vi "Turbulence_3.0_LevelResistors.vi"() -> ()   [LabVIEW 2018]
uses:
  Quantum Composers 9000 Series.lvlib
  LightField Automation.lvclass
  Mercury iXX.lvlib
  Temperature (Read).vi
  Temperature.lvlib
  Open Temperature Device.vi
  Comms Transport Layer.ctl
  Keithley 2600 Series.lvlib
  Channel.ctl
  DAQmx Read (Counter DBL 1Chan 1Samp).vi
  Catalogue (Read).vi
  System.lvlib
  Open System.vi
panel:
  in  "3He Check":bool
  out "MFC Error Out":errorcluster
  out "Lakeshore218 Error":errorcluster
  in  "File Exists":bool
  out "Log":refnum<file>
  in  "Motor free":bool
  in  "RESTART":bool
  out "time string":string
  out "Timestamp":string
  out "Log Error":errorcluster
  in  "CLOSE":bool
  in  "RECORD":bool
  in  "Turbulence":T1(tab)
  in  "# Frames":i32=1000 min=0 step=1
  in  "New Background Movie":bool
  in  "On CCD Acc.":i32=3 min=0 step=1
  in  "Cycle time\n(ms)":i32=3 min=0 step=1
  out "High Level\n(Ohms)":dbl format="%.1f"
  out "Low Level\n(Ohms)":dbl format="%.1f"
  in  "New Background Frame":bool
  out "Rate (Hz)":dbl
  out "Incident":dbl
  in  "BIN":u16(ring)=2 items=["1x1", "2x2", "4x4"]
  in  "MODE":u16(ring) items=["Normal", "DIF"]
  in  "Enable":bool
  out "Rate (Hz)":dbl
  out "Detected":dbl
  in  "Script\nEnd":u32=1 step=1
  in  "Sample Space Pump":bool
  in  "Siphon Pump":bool
  in  "Neutron Shutter":bool
  in  "Manual Script Entry (0)":string
  in  "READY":bool
  out "Power (mW)":dbl format="%_3f"
  out "Tank Pressure 2 (Torr)":string="0.0"
  in  "LIGHTFIELD":bool
  in  "SCRIPTING":bool
  in  "Top Coil":bool
  out "Tank Pressure 1 (Torr)":string="0.0"
  out "Cell (K)":dbl format="%.3f"
  out "Cryostat (K)":dbl format="%.3f"
  in  "Data Interval (s)":dbl=0.5 min=0.4 max=10.0 step=0.05
  in  "RUN/STOP":bool
  in  "Bottom Coil":bool
  in  "Bottom Coil (mA)":dbl min=-1000.0 max=1000.0 step=1e-05
  in  "Top Coil (mA)":dbl min=-1000.0 max=1000.0 step=1e-05
  in  "Percent Open":i32 min=0 max=100 step=5
  in  "COOLDOWN":bool
  in  "Script\n#":i32 step=1
  in  "Kill Switch":bool
  in  "DATA":bool
  out "Scripting \nError":T2
  in  "Shutter Mode":u16(ring)=1 items=["Manual"=1, "XGate"=5]
  in  "Time (s)":i32=120 min=1 max=300 step=1
  in  "REFILL":bool
  in  "AUTOFILL":bool
  in  "LL (Ohms)":dbl=900.0 min=750.0 max=15000.0 step=1.0
  in  "HL (Ohms)":dbl=900.0 min=750.0 max=15000.0 step=1.0
  in  "Fill":bool
  in  "Tare":bool
  out "Actual 3He\nTank Pressure":dbl min=0.0 max=100.0 step=5.0 format="%#.1g"
  out "Desired V2\nPressure (3He)":dbl min=0.0 max=100.0 step=5.0 format="%#.1f"
  in  "Desired Tank\nPressure (3He)":dbl min=0.0 max=100.0 step=0.01 format="%#.2f"
  in  "Log Pressure":bool
  out "4He Pressure (Torr)":string="-0.1"
  out "3He Pressure (Torr)":string="1"
  in  "Fill Time (s)":u32=10
  out "Temperature Error":errorcluster={"status"=TRUE, "code"=-1073807339, "source"="VISA Read in Mercury iXX.lvlib:Query (Dynamic).vit->Mercury iXX.lvlib:Query (Low Level).vi:10049->Mercury iXX.lvlib:Query.vi:3960048->Mercury iXX.lvlib:Read (Str).vi:5300004->Mercury iXX.lvlib:System.lvlib:Catalogue (Read).vi->Turbulence.vi"}
  out "File I/O Error":errorcluster
  out "4He Gauge Error":errorcluster={"status"=TRUE, "code"=-1073807343, "source"="VISA Open in Turbulence.vi"}
  out "Heater Error":errorcluster={"status"=FALSE, "code"=1073676293, "source"="VISA Read in Keithley 2600 Series.lvlib:Print Number.vi->Keithley 2600 Series.lvlib:Measure.vi->Turbulence.vi"}
  out "Pulse Generator Error":errorcluster
  out "3He Gauge Error":errorcluster={"status"=FALSE, "code"=1073676293, "source"="VISA Read in 3HeClose.vi->Turbulence.vi"}
  out "Relay Errror":errorcluster
  out "Zaber Motor Error":errorcluster
  out "LightField Error":errorcluster
  out "Shutter Error":errorcluster
  # "Camera Controls"
  # "Temperature Readout"
  # "Pressure Readout"
  # "Neutron Counts"
  # "Automation"
  # "Heater Controls"
  # "Relay Controls"
  # "Needle Valve Control"
  # "Neutron Shutter"
  # "Optical Shutter"
  # "Siphon Pump"
  # "Laser Power Meter"
  # "Sample Space\nPump"
  # "V1 = 4075 mL"
  # "V2 = 15.5 mL"
  # "V3 = 78.8 mL"
  # "Quartz\nCell"
  # "4"
  # "3psi relief"
  # "MFC"
  # "V1"
  # "4L Tank"
  # "Turbo Pump"
  # "V2"
  # "V3"
  # "3"
  # "10psi relief"
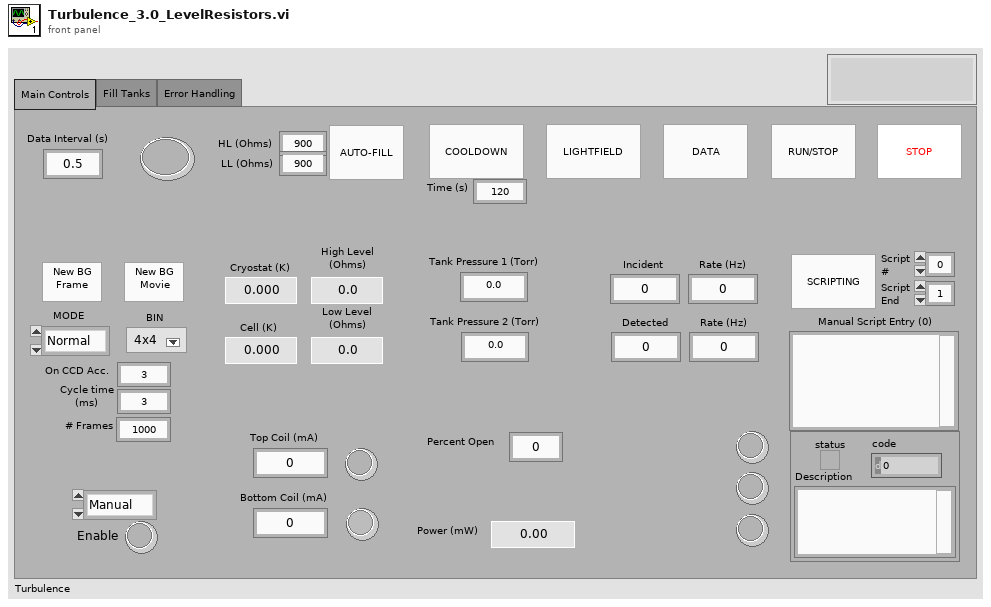
[diagram p1: front panel]
types:
  T1 = enum32{"Main Controls", "Fill Tanks", "Error Handling"}
  T2 = cluster{"status":bool, "code":i32, "Description":string}
  T3 = typedef "Mercury iXX.lvlib/Comms Transport Layer.ctl" = enum16{"Ethernet TCP/IP", "USB", "ISOBus - RS-232", "GPIB"}
  T4 = typedef "Mercury iXX.lvlib/Mercury Reference.ctl" = cluster{"Comms":refnum<visa-resource-name>, "Device ID":string[], "Comms Layer":T3, "Command":string, "Query reference":T5}
  T5 = typedef "Mercury iXX.lvlib/Query Dynamic Reference.ctl" = refnum<vi>
  T6 = enum32{"Current", "Voltage", "IV", "Resistance", "Power"}
  T7 = typedef "Keithley 2600 Series.lvlib/Channel.ctl" = enum32{"Channel A", "Channel B"}
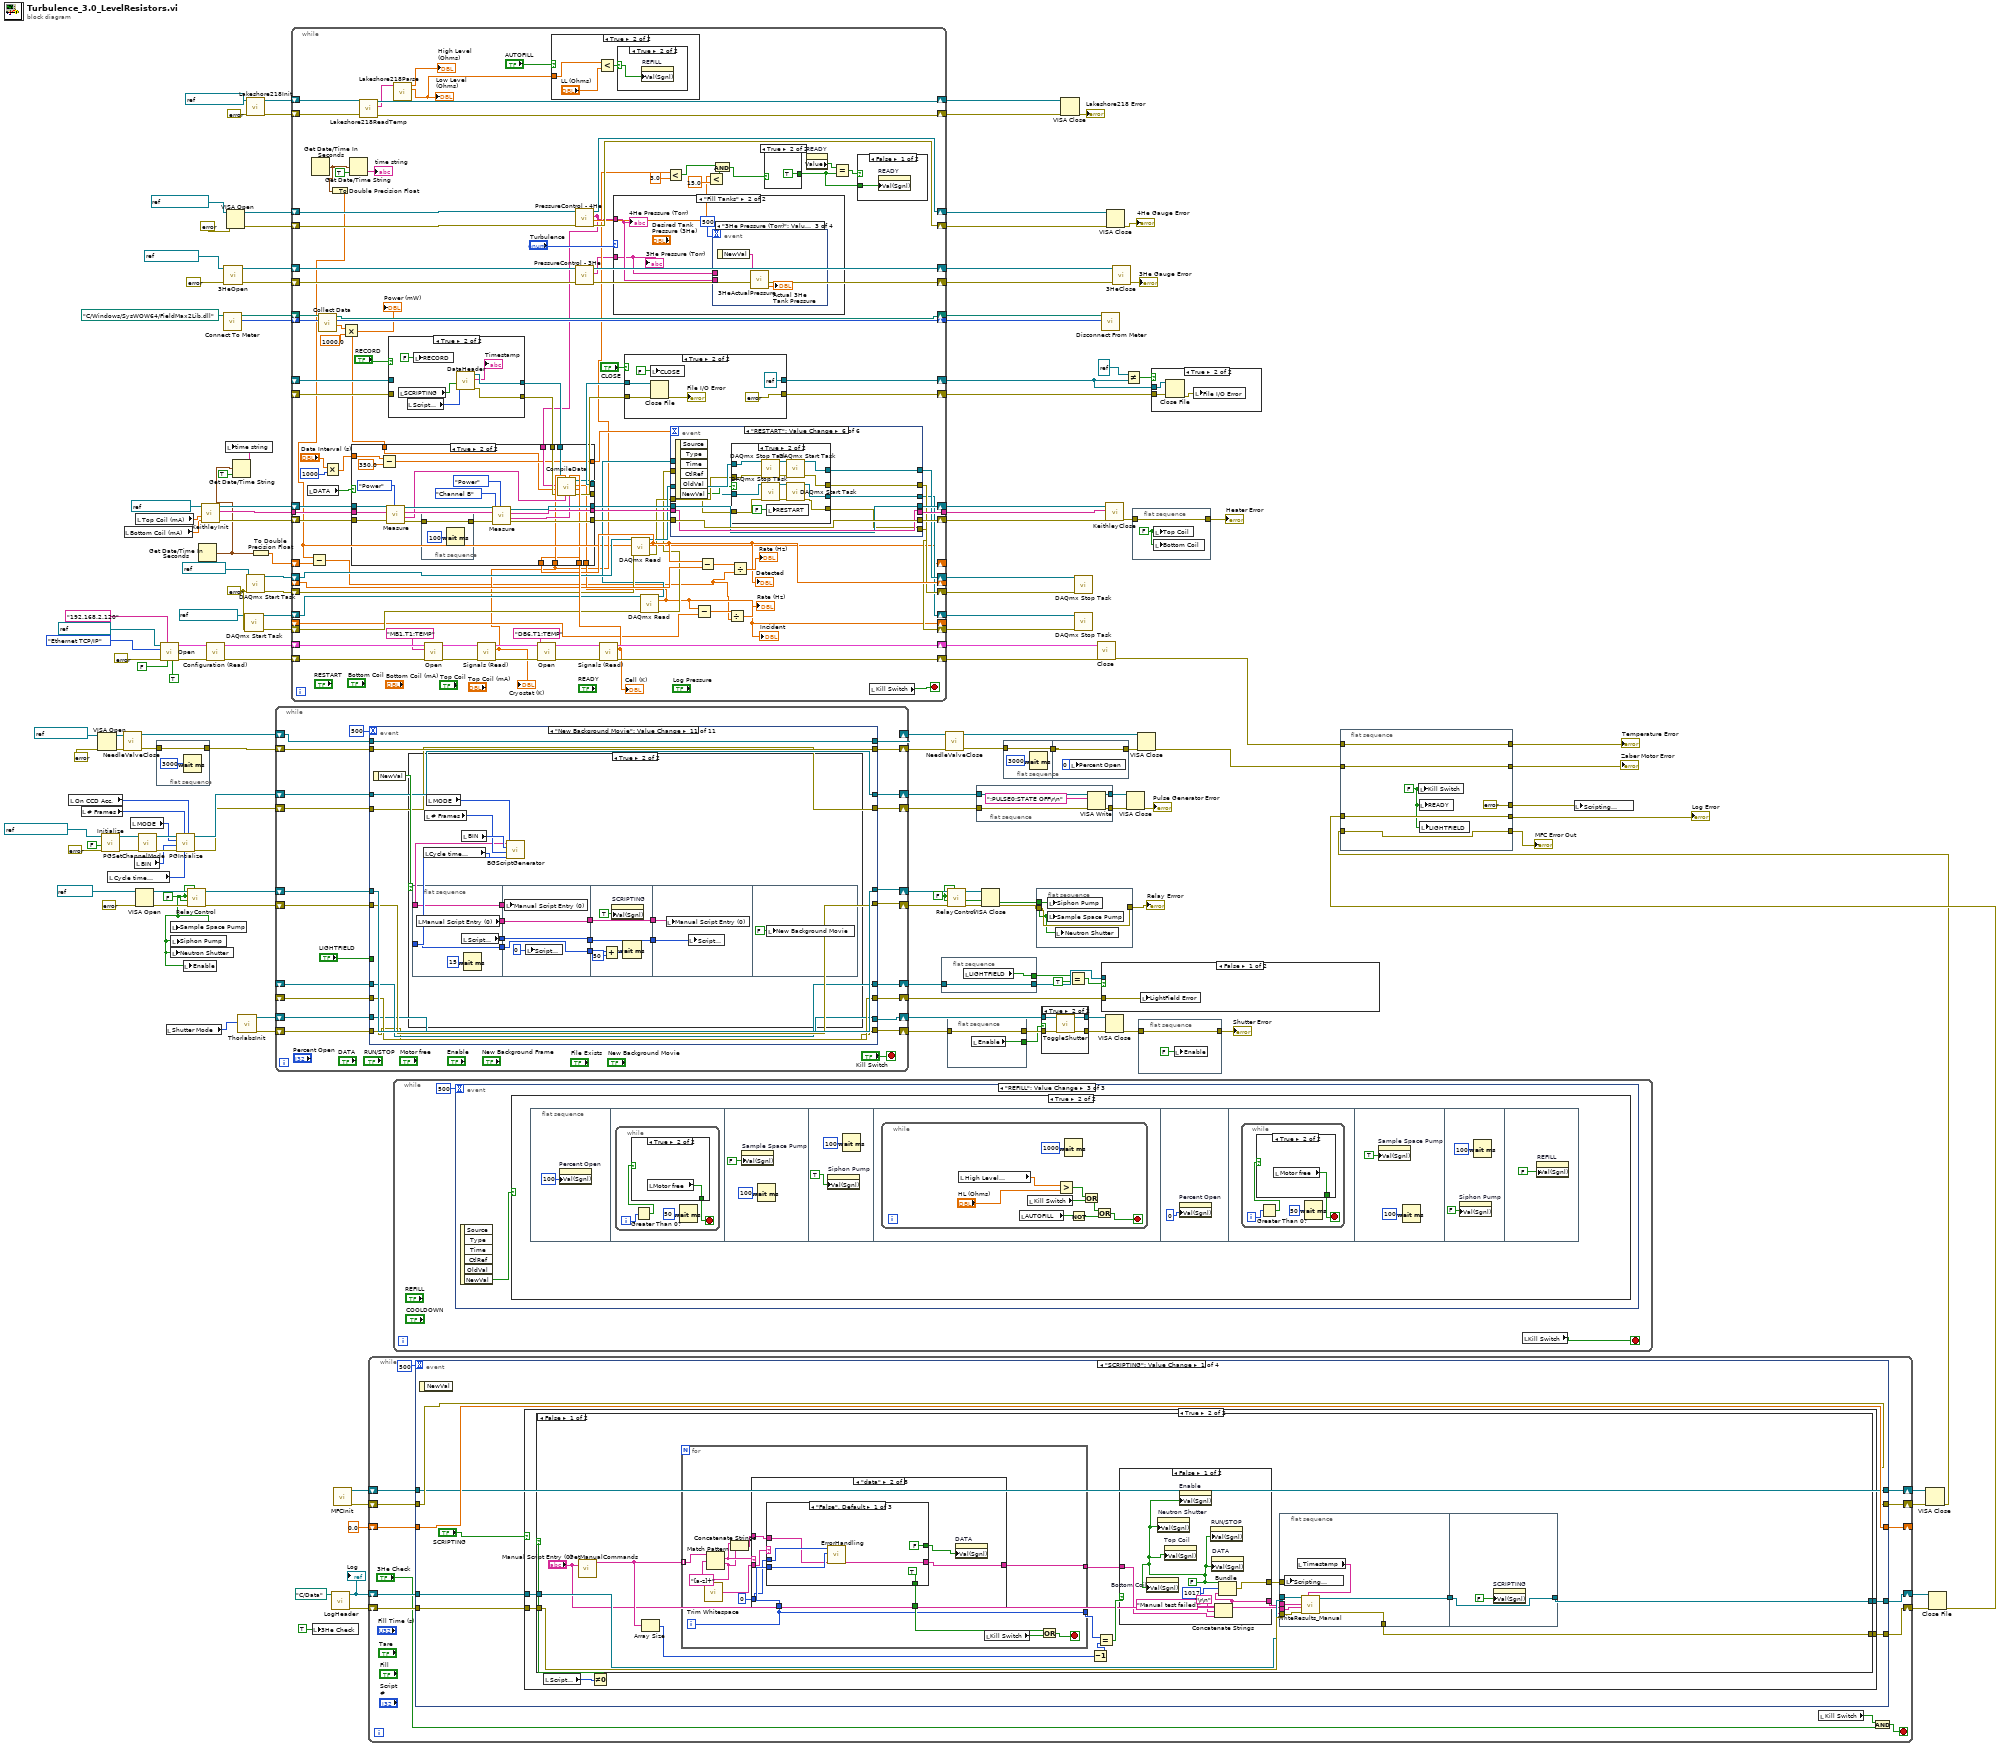
[diagram p0: block diagram]
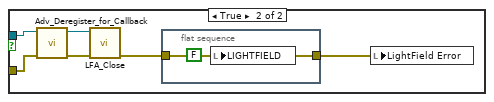
[diagram p3: hidden frame]
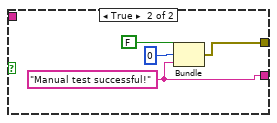
[diagram p5: hidden frame]
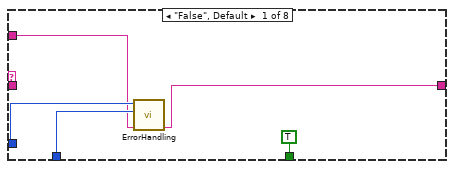
[diagram p6: hidden frame]
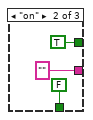
[diagram p7: hidden frame]
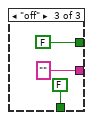
[diagram p8: hidden frame]
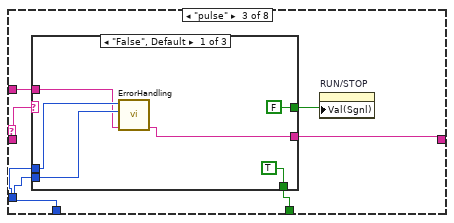
[diagram p9: hidden frame]
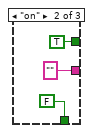
[diagram p10: hidden frame]
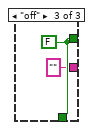
[diagram p11: hidden frame]
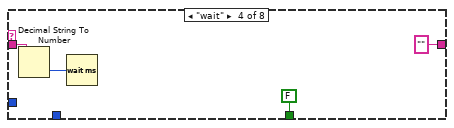
[diagram p12: hidden frame]
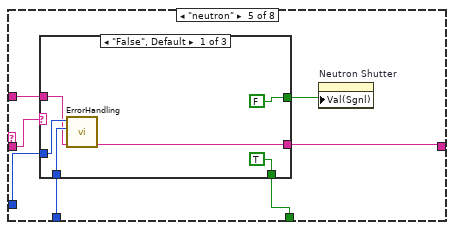
[diagram p13: hidden frame]
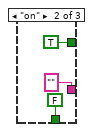
[diagram p14: hidden frame]
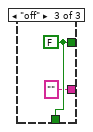
[diagram p15: hidden frame]
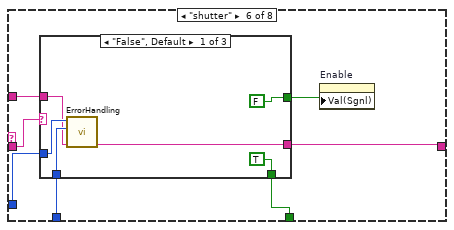
[diagram p16: hidden frame]
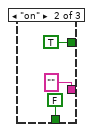
[diagram p17: hidden frame]
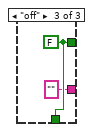
[diagram p18: hidden frame]
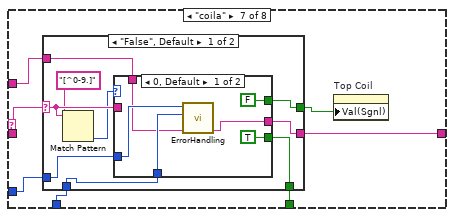
[diagram p19: hidden frame]
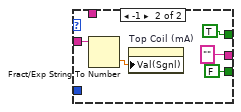
[diagram p20: hidden frame]
diagram:
  w39 = errorcluster {"status"=FALSE, "code"=0, "source"=""} ("error in")
  w76 = FALSE ("Siphon Pump")
  w61 = FALSE ("Siphon Pump")
  n1 = local read "On CCD Acc."() -> (w50:i32)
  n2 = local read "# Frames"() -> (w49:i32)
  n3 = VISA Open(error in (no error)=errorcluster {"status"=FALSE, "code"=0, "source"=""}, VISA resource name=refnum<visa-resource-name> "ZaberMotor") -> (VISA resource name=w56:refnum<visa-resource-name>, error out=w57:errorcluster)  [unwired: 3 in]
  n4 = call "Initialize.vi"("error in (no error)"=errorcluster {"status"=FALSE, "code"=0, "source"=""}, "Reset? (T: Yes)"=FALSE, "VISA resource name"=refnum<visa-resource-name> "PulseGenerator" ("Pulse generater (COM3)")) -> ("error out"=w68:errorcluster, "VISA resource name out"=w66:refnum<visa-resource-name>)  [unwired: 7 in]
  n5 = local read "Cycle time\n(ms)"() -> (w10:i32)
  n6 = call "NeedleValveClose.vi"("error in (no error)"=w57, "VISA resource name"=w56) -> ("error out"=w58:errorcluster, "VISA resource name out"=w98:refnum<visa-resource-name>)  [unwired: 8 in]
  n7 = local read "Bottom Coil (mA)"() -> (w110:dbl)
  n8 = local read "MODE"() -> (w47:u16)
  n9 = local read "BIN"() -> (w48:u16)
  n10 = VISA Open(error in (no error)=errorcluster {"status"=FALSE, "code"=0, "source"=""} ("error in (no error) 2"), VISA resource name=refnum<visa-resource-name> "Relays" ("Pressure Gauge")) -> (VISA resource name=w123:refnum<visa-resource-name>, error out=w125:errorcluster)  [unwired: 3 in]
  n11 = local read "Top Coil (mA)"() -> (w111:dbl)
  n12 = call "PGSetChannelMode.vi"("error in"=w68, "VISA resource name"=w66) -> ("error out"=w67:errorcluster, "VISA resource name out"=w65:refnum<visa-resource-name>)  [unwired: 8 in]
  n13 = flat-sequence {
    tunnel: w58 -> [w152]
    tunnel: [w152] -> w99
    frame #0 {
      n14 = Wait (ms)(milliseconds to wait=u32 3000) -> ()  [unwired: 1 out]
    }
  }
  n15 = call-poly "Open.vi"("Clear Previous Connections (False)"=TRUE, "ID Query (True)"=FALSE, "IP Address"="192.168.2.120", "error in (no error)"=errorcluster {"status"=FALSE, "code"=0, "source"=""}, "Comms Layer"=Comms_Transport_Layer."Ethernet TCP/IP", "VISA resource name"=refnum<visa-resource-name> "MercuryiTC") -> ("error out"=w144:errorcluster, "Mercury Reference Out"=w145:T4)  [unwired: 1 in, 3 out]
  n16 = local read "Shutter Mode"() -> (w51:u16)
  n17 = local write "Sample Space Pump"(w61) -> ()
  n18 = local write "Neutron Shutter"(w61) -> ()
  n19 = local write "Siphon Pump"(w61) -> ()
  n20 = call "PGIntialize.vi"("On CCD Accumulations"=w50, "Cycle time\n(ms)"=w10, "Number of Frames"=w49, "error in"=w67, "BIN"=w48, "MODE"=w47, "VISA resource name"=w65) -> ("error out"=w149:errorcluster, "VISA resource name out"=w150:refnum<visa-resource-name>)  [unwired: 3 in]
  n21 = local write "Enable"(w61) -> ()
  n22 = call "RelayControl.vi"("Neutron Shutter"=w61, "Error In"=w125, "Sample Space Pump"=w61, "Siphon Pump"=w61, "Relay In"=w123) -> ("Error Out"=w124:errorcluster, "Relay Out"=w122:refnum<visa-resource-name>)  [unwired: 5 in]
  n23 = Get Date/Time In Seconds() -> (seconds since 1Jan1904=w18:timestamp)
  n24 = call "KeithleyInit.vi"("Bottom Coil (mA)"=w110, "Top Coil (mA)"=w111, "KeithleyVISA In"=refnum<visa-resource-name> "Keithley2614B" ("VISA resource name")) -> ("error out"=w114:errorcluster, "Node Out"=w115:string, "KeithleyVISA Out"=w113:refnum<visa-resource-name>)  [unwired: 6 in]
  n25 = call-poly "Configuration (Read).vi"("error in"=w144, "Mercury Reference In"=w145) -> ("error out"=w140:errorcluster, "Mercury Reference Out"=w141:T4)  [unwired: 6 in, 2 out]
  n26 = call "Connect To Meter.vi"("Location of FieldMax2Lib.dll in"=path "C:/Windows/SysWOW64/FieldMax2Lib.dll") -> ("Meter ID out"=w84:i32, "Location of FieldMax2Lib.dll out"=w83:path)  [unwired: 6 in, 1 out]
  n27 = call "3HeOpen.vi"("error in (no error)"=errorcluster {"status"=FALSE, "code"=0, "source"=""} ("error in (no error) 2"), "VISA resource name"=refnum<visa-resource-name> "3HePressure" ("Pressure Gauge")) -> ("error out"=w127:errorcluster, "VISA resource name out"=w126:refnum<visa-resource-name>)  [unwired: 8 in]
  n28 = VISA Open(error in (no error)=errorcluster {"status"=FALSE, "code"=0, "source"=""} ("error in (no error) 2"), VISA resource name=refnum<visa-resource-name> "TankPressure" ("Pressure Gauge")) -> (VISA resource name=w137:refnum<visa-resource-name>, error out=w138:errorcluster)  [unwired: 3 in]
  n29 = Get Date/Time String(seconds (now)=w18, want seconds? (F)=TRUE) -> (time string=w19:string)  [unwired: 1 in, 1 out]
  n30 = local write "time string"(w19) -> ()
  n31 = call "ThorlabsInit.vi"("Shutter Mode"=w51) -> ("error out"=w62:errorcluster, "VISA resource name out"=w63:refnum<visa-resource-name>)  [unwired: 9 in]
  n32 = call "DAQmx Start Task.vi"("task/channels in"=refnum<k21> "IncidentBeam", "error in"=w39) -> ("task out"=w41:refnum<k21>, "error out"=w40:errorcluster)  [unwired: 12 in]
  n33 = call "Lakeshore218Init.vi"("error in (no error)"=errorcluster {"status"=FALSE, "code"=0, "source"=""}, "VISA resource name"=refnum<visa-resource-name> "Lakeshore218") -> ("error out"=w16:errorcluster, "VISA resource name out"=w15:refnum<visa-resource-name>)  [unwired: 8 in]
  n34 = call "DAQmx Start Task.vi"("task/channels in"=refnum<k21> "Detector", "error in"=w39) -> ("task out"=w44:refnum<k21>, "error out"=w43:errorcluster)  [unwired: 12 in]
  n35 = To Double Precision Float(number=w18) -> (double precision float=w21:dbl)
  n36 = while {
    shift-right: [w175] -> w28
    shift-left: _ -> [w173]
    shift-right: [w176] -> w35
    shift-left: _ -> [w174]
    shift-right: [w169] -> w92
    shift-left: w150 -> [w171]
    shift-right: [w170] -> w93
    shift-left: w149 -> [w172]
    shift-right: [w165] -> w97
    shift-left: w124 -> [w168]
    shift-right: [w166] -> w95
    shift-left: w122 -> [w167]
    shift-right: [w160] -> w128
    shift-left: w99 -> [w163]
    shift-right: [w161] -> w129
    shift-left: w98 -> [w162]
    shift-right: [w157] -> w31
    shift-left: w63 -> [w154]
    shift-right: [w156] -> w24
    shift-left: w62 -> [w155]
    stop <- "Kill Switch" stop-if-true
    n37 = event shown="[10] \"New Background Movie\": Value Change" {
      selector: _ -> [_ _ _ _ _ _ _ _ _ _ _]
      dyn-events: _ -> [_ _ _ _ _ _ _ _ _ _ _]
      timeout: 500 -> [_ _ _ _ _ _ _ _ _ _ _]
      tunnel: w172 -> [w184 w193 w270 w316 w334 w382 w447 w466 w481 w504 w528]
      tunnel: w171 -> [w183 w192 w271 w317 w333 w383 w448 w465 w480 w503 w529]
      tunnel: w174 -> [w185 w196 w261 w308 w336 w386 w445 w469 w485 w495 w524]
      tunnel: w173 -> [w186 w197 w262 w309 w337 w387 w446 w470 w484 w496 w525]
      tunnel: [w185 w198 w260 w308 w336 w374 w445 w469 w485 w495 w524] -> w176
      tunnel: [w186 w199 w259 w309 w337 w366 w446 w470 w484 w496 w525] -> w175
      tunnel: [w184 w193 w273 w316 w334 w372 w447 w466 w481 w501 w528] -> w170
      tunnel: [w183 w192 w272 w317 w333 w379 w448 w465 w480 w502 w529] -> w169
      tunnel: w168 -> [w181 w194 w267 w314 w339 w381 w454 w468 w483 w497 w526]
      tunnel: w167 -> [w182 w195 w268 w315 w338 w380 w453 w467 w482 w498 w527]
      tunnel: [w182 w195 w268 w315 w338 w380 w450 w467 w482 w498 w527] -> w166
      tunnel: [w181 w194 w267 w314 w339 w381 w449 w468 w483 w497 w526] -> w165
      tunnel: w163 -> [w180 w191 w266 w318 w322 w385 w444 w464 w479 w499 w530]
      tunnel: w162 -> [w179 w190 w265 w319 w335 w384 w443 w463 w478 w500 w531]
      tunnel: [w179 w190 w265 w319 w332 w384 w443 w463 w478 w500 w531] -> w161
      tunnel: [w180 w191 w266 w318 w324 w385 w444 w464 w479 w499 w530] -> w160
      tunnel: "LIGHTFIELD" -> [_ _ w258 w313 _ w368 _ _ _ w491 _]
      tunnel: w154 -> [w177 w188 w264 w311 w330 w378 w441 w462 w489 w494 w523]
      tunnel: w155 -> [w178 w187 w263 w310 w329 w377 w440 w461 w488 w493 w522]
      tunnel: [w177 w188 w264 w311 w330 w378 w441 w459 w486 w494 w523] -> w157
      tunnel: [w178 w187 w263 w310 w329 w377 w440 w460 w487 w493 w522] -> w156
      event Timeout {
        n38 = event-data() -> ()  [unwired: 1 in, 3 out]
      }
      event "LIGHTFIELD": Value Change {
        n39 = event-data() -> ("NewVal"=w189:bool)  [unwired: 1 in, 5 out]
        n40 = case shown="True" w189 {
          tunnel: [refnum<class "LightField Automation.lvclass"> refnum ("LightField Automation out") w215] -> w199
          tunnel: [errorcluster {"status"=FALSE, "code"=0, "source"=""} ("error out") w214] -> w198
          tunnel: w197 -> [w203 _]
          tunnel: w196 -> [w202 _]
          frame False {
            n41 = call "Adv_Deregister_for_Callback.vi"("error in (no error)"=w202, "LightField Automation in"=w203) -> ("error out"=w205:errorcluster, "LightField Automation out"=w206:refnum<class "LightField Automation.lvclass">)  [unwired: 8 in]
            n42 = call "LFA_Close.vi"("error in (no error)"=w205, "LightField Automation in"=w206) -> ("error out"=→"LightField Error":errorcluster)  [unwired: 8 in, 1 out]
          }
          frame True {
            n43 = call "LFA_Initialize.vi"("error in (no error)"=errorcluster {"status"=FALSE, "code"=0, "source"=""}) -> ("error out"=w224:errorcluster, "LightField Automation out"=w223:refnum<class "LightField Automation.lvclass">)  [unwired: 9 in]
            n44 = call "Adv_Register_for_Callback.vi"("error in (no error)"=w224, "LightField Automation in"=w223) -> ("error out"=w222:errorcluster, "LightField Automation out"=w221:refnum<class "LightField Automation.lvclass">)  [unwired: 8 in]
            n45 = call "Exp_SetExperiment.vi"("error in (no error)"=w222, "ExperimentName"="20190801_DIF", "LightField Automation in"=w221) -> ("error out"=w208:errorcluster, "LightField Automation out"=w207:refnum<class "LightField Automation.lvclass">)  [unwired: 7 in]
            n46 = flat-sequence {
              tunnel: [w228] -> w212
              tunnel: [w227] -> w211
              tunnel: [w226] -> w210
              tunnel: [w229] -> w209
              tunnel: w208 -> [w232]
              tunnel: w207 -> [w230]
              tunnel: [w243] -> w218
              tunnel: [w242] -> w217
              tunnel: [w241] -> w216
              tunnel: [w240] -> w213
              tunnel: w212 -> [w240]
              tunnel: w211 -> [w243]
              tunnel: w210 -> [w242]
              tunnel: w209 -> [w241]
              tunnel: w218 -> [w248]
              tunnel: w217 -> [w249]
              tunnel: w216 -> [w247]
              tunnel: [w246] -> w215
              tunnel: [w245] -> w214
              tunnel: w213 -> [w244]
              frame #0 {
                n47 = local read "On CCD Acc."() -> (w238:i32)
                n48 = local read "Cycle time\n(ms)"() -> (w225:i32)
                n49 = local read "# Frames"() -> (w236:i32)
                n50 = local read "BIN"() -> (w237:u16)
                n51 = call "Exp_ICCD_SetIntensifierGain.vi"("error in (no error)"=w232, "Intensifier Gain"=100, "LightField Automation in"=w230) -> ("error out"=w234:errorcluster, "LightField Automation out"=w233:refnum<class "LightField Automation.lvclass">)  [unwired: 7 in]
                n52 = local read "MODE"() -> (w239:u16)
                n53 = local read "Log"() -> (w235:refnum<file>)
                n54 = call "LightFieldInit.vi"("On CCD Accumulations"=w238, "File Path"=w235, "Number of Frames"=w236, "error in"=w234, "BIN"=w237, "MODE"=w239, "LightField Automation in"=w233) -> ("error out"=w227:errorcluster, "LightField Automation out"=w226:refnum<class "LightField Automation.lvclass">)  [unwired: 3 in]
                n55 = call "LightFieldBackgroundNaming.vi"("Cycle time\n(ms)"=w225, "On CCD Acc."=w238, "BIN"=w237, "MODE"=w239) -> ("FilePath"=w229:string, "Exists"=w228:bool)  [unwired: 5 in, 1 out]
              }
              frame #1 {
                n56 = local write "File Exists"(w240) -> ()
              }
              frame #2 {
                n57 = case shown="False" w244 {
                  tunnel: w249 -> [w252 w257]
                  tunnel: w248 -> [w251 w256]
                  tunnel: w247 -> [_ w255]
                  tunnel: [w252 w254] -> w246
                  tunnel: [w251 w253] -> w245
                  frame False {
                    n58 = property on="New Background Frame" class="Bool (strict)"("Val(Sgnl)"=TRUE ("Value (Signaling)")) -> ()  [unwired: 2 in, 2 out]
                  }
                  frame True {
                    n59 = call "LightFieldChangeBackground.vi"("error in"=w256, "FilePath"=w255, "LightField Automation in"=w257) -> ("error out"=w253:errorcluster, "LightField Automation out"=w254:refnum<class "LightField Automation.lvclass">)  [unwired: 7 in]
                  }
                }
              }
            }
          }
        }
      }
      event "RUN/STOP": Value Change {
        n60 = event-data() -> ("NewVal"=w269:bool)  [unwired: 1 in, 5 out]
        n61 = case shown="True" w269 {
          tunnel: [w277 w290] -> w273
          tunnel: [w278 w289] -> w272
          tunnel: w271 -> [w279 w288]
          tunnel: w270 -> [w280 w287]
          tunnel: w262 -> [w275 w285]
          tunnel: w261 -> [w274 w284]
          tunnel: [w274 w283] -> w260
          tunnel: [w275 w282] -> w259
          tunnel: w258 -> [_ w281]
          frame False {
            n62 = VISA Write(VISA resource name=w279, write buffer=":PULSE0:STATE OFF\r\n" ("format string"), error in (no error)=w280) -> (VISA resource name out=w278:refnum<visa-resource-name>, error out=w277:errorcluster)  [unwired: 1 out]
          }
          frame True {
            n63 = case shown="True" w281 {
              tunnel: w284 -> [w291 w303]
              tunnel: w285 -> [w292 w301]
              tunnel: [w292 w305] -> w282
              tunnel: [w291 w304] -> w283
              frame False {
              }
              frame True {
                n64 = local read "New Background Movie"() -> (w295:bool)
                n65 = local read "Cycle time\n(ms)"() -> (w293:i32)
                n66 = local read "On CCD Acc."() -> (w294:i32)
                n67 = local read "MODE"() -> (w298:u16)
                n68 = local read "SCRIPTING"() -> (w296:bool)
                n69 = local read "BIN"() -> (w299:u16)
                n70 = case shown="True" w296 {
                  tunnel: [-1 ("Script\n#") w307] -> w297
                  frame False {
                  }
                  frame True {
                    n71 = local read "Script\n#"() -> (w307:i32)
                  }
                }
                n72 = call "LightFieldFileNaming.vi"("Cycle time\n(ms)"=w293, "On CCD Acc."=w294, "Script#"=w297, "BG"=w295, "error in"=w303, "BIN"=w299, "MODE"=w298, "LightField Automation in"=w301) -> ("error out"=w302:errorcluster, "LightField Automation out"=w300:refnum<class "LightField Automation.lvclass">)  [unwired: 2 in]
                n73 = call "LFA_Acquire.vi"("error in (no error)"=w302, "LightField Automation in"=w300) -> ("error out"=w304:errorcluster, "LightField Automation out"=w305:refnum<class "LightField Automation.lvclass">)  [unwired: 8 in]
              }
            }
            n74 = VISA Write(VISA resource name=w288, write buffer=":PULSE0:STATE ON\r\n" ("format string"), error in (no error)=w287) -> (VISA resource name out=w289:refnum<visa-resource-name>, error out=w290:errorcluster)  [unwired: 1 out]
          }
        }
      }
      event "DATA": Value Change {
        n75 = event-data() -> ("NewVal"=w312:bool)  [unwired: 1 in, 5 out]
        n76 = case shown="False" w312 {
          tunnel: w313 -> [_ _]
          frame False {
            n77 = local write "CLOSE"(TRUE ("CLOSE")) -> ()
          }
          frame True {
            n78 = local write "RECORD"(TRUE ("RECORD")) -> ()
          }
        }
      }
      event "Percent Open": Value Change {
        n79 = event-data() -> ("OldVal"=w331:i32, "NewVal"=w340:i32)  [unwired: 1 in, 4 out]
        n80 = flat-sequence {
          tunnel: w322 -> [w342]
          tunnel: [w342] -> w323
          frame #0 {
            n81 = property on="Motor free" class="Bool (strict)"("Val(Sgnl)"=FALSE ("Value (Signaling)")) -> ()  [unwired: 2 in, 2 out]
          }
        }
        n82 = Subtract(x=w340, y=w331) -> (x-y=w326:i32)
        n83 = Greater Than 0?(x=w326) -> (x > 0?=w327:bool)
        n84 = Equal To 0?(x=w340) -> (x = 0?=w328:bool)
        n85 = case shown="False" w328 {
          tunnel: w335 -> [w348 w364]
          tunnel: w323 -> [w349 w363]
          tunnel: [w347 w362] -> w332
          tunnel: [w346 w361] -> w325
          tunnel: w327 -> [w350 _]
          tunnel: w326 -> [w345 _]
          frame False {
            n86 = case shown="True" w350 {
              tunnel: w349 -> [w354 w360]
              tunnel: w348 -> [w355 w359]
              tunnel: [w353 w358] -> w347
              tunnel: [w352 w357] -> w346
              tunnel: w345 -> [w351 w356]
              frame False {
                n87 = call "NeedleValveClose - Encoder.vi"("error in (no error)"=w354, "Percent Difference"=w351, "VISA resource name"=w355) -> ("error out"=w352:errorcluster, "VISA resource name out"=w353:refnum<visa-resource-name>)  [unwired: 7 in]
              }
              frame True {
                n88 = call "NeedleValveOpen - Encoder.vi"("error in (no error)"=w360, "Percent Difference"=w356, "VISA resource name"=w359) -> ("error out"=w357:errorcluster, "VISA resource name out"=w358:refnum<visa-resource-name>)  [unwired: 7 in]
              }
            }
          }
          frame True {
            n89 = call "NeedleValveClose.vi"("error in (no error)"=w363, "VISA resource name"=w364) -> ("error out"=w361:errorcluster, "VISA resource name out"=w362:refnum<visa-resource-name>)  [unwired: 8 in]
          }
        }
        n90 = flat-sequence {
          tunnel: w325 -> [w344]
          tunnel: [w344] -> w324
          frame #0 {
            n91 = property on="Motor free" class="Bool (strict)"("Val(Sgnl)"=TRUE ("Value (Signaling)")) -> ()  [unwired: 2 in, 2 out]
          }
        }
      }
      event "Cycle time\n(ms)", "# Frames", "MODE", "BIN", "On CCD Acc.": Value Change {
        n92 = event-data() -> ()  [unwired: 1 in, 1 out]
        n93 = case shown="True" w368 {
          tunnel: w387 -> [w428 w436]
          tunnel: w386 -> [w429 w437]
          tunnel: [w428 w435] -> w367
          tunnel: [w429 w434] -> w375
          tunnel: "On CCD Acc." -> [_ w432]
          tunnel: "# Frames" -> [_ w433]
          tunnel: "BIN" -> [_ w431]
          tunnel: "MODE" -> [_ w430]
          frame False {
          }
          frame True {
            n94 = call "LightFieldParams.vi"("On CCD Accumulations"=w432, "Number of Frames"=w433, "error in"=w437, "BIN"=w431, "MODE"=w430, "LightField Automation in"=w436) -> ("error out"=w434:errorcluster, "LightField Automation out"=w435:refnum<class "LightField Automation.lvclass">)  [unwired: 4 in]
          }
        }
        n95 = call "PGIntialize.vi"("On CCD Accumulations"="On CCD Acc.", "Cycle time\n(ms)"="Cycle time\n(ms)", "Number of Frames"="# Frames", "error in"=w382, "BIN"="BIN", "MODE"="MODE", "VISA resource name"=w383) -> ("error out"=w373:errorcluster, "VISA resource name out"=w379:refnum<visa-resource-name>)  [unwired: 3 in]
        n96 = case shown="True" w368 {
          tunnel: w375 -> [w390 w400]
          tunnel: [w390 w399] -> w374
          tunnel: w373 -> [w389 w398]
          tunnel: [w389 w397] -> w372
          tunnel: "On CCD Acc." -> [_ w396]
          tunnel: "BIN" -> [_ w395]
          tunnel: "MODE" -> [_ w394]
          tunnel: w367 -> [w388 w393]
          tunnel: [w388 w392] -> w366
          tunnel: "Cycle time\n(ms)" -> [_ w391]
          frame False {
          }
          frame True {
            n97 = flat-sequence {
              tunnel: w400 -> [w404]
              tunnel: [w403] -> w399
              tunnel: w398 -> [w412]
              tunnel: [w412] -> w397
              tunnel: w396 -> [w411]
              tunnel: w395 -> [w410]
              tunnel: w394 -> [w409]
              tunnel: w393 -> [w405]
              tunnel: [w402] -> w392
              tunnel: w391 -> [w401]
              frame #0 {
                n98 = call "LightFieldBackgroundNaming.vi"("Cycle time\n(ms)"=w401, "On CCD Acc."=w411, "BIN"=w410, "MODE"=w409) -> ("FilePath"=w406:string, "Exists"=w408:bool)  [unwired: 5 in, 1 out]
                n99 = flat-sequence {
                  tunnel: w408 -> [w413]
                  tunnel: [w413] -> w407
                  tunnel: w407 -> [w419]
                  tunnel: w406 -> [w418]
                  tunnel: w405 -> [w417]
                  tunnel: w404 -> [w416]
                  tunnel: [w415] -> w403
                  tunnel: [w414] -> w402
                  frame #0 {
                    n100 = local write "File Exists"(w413) -> ()
                  }
                  frame #1 {
                    n101 = case shown="True" w419 {
                      tunnel: w418 -> [_ w427]
                      tunnel: w417 -> [w421 w426]
                      tunnel: w416 -> [w420 w425]
                      tunnel: [w420 w424] -> w415
                      tunnel: [w421 w423] -> w414
                      frame False {
                        n102 = property on="New Background Frame" class="Bool (strict)"("Val(Sgnl)"=TRUE ("Value (Signaling)")) -> ()  [unwired: 2 in, 2 out]
                      }
                      frame True {
                        n103 = call "LightFieldChangeBackground.vi"("error in"=w425, "FilePath"=w427, "LightField Automation in"=w426) -> ("error out"=w424:errorcluster, "LightField Automation out"=w423:refnum<class "LightField Automation.lvclass">)  [unwired: 7 in]
                      }
                    }
                  }
                }
              }
            }
          }
        }
      }
      event "Siphon Pump", "Sample Space Pump", "Neutron Shutter": Value Change {
        n104 = event-data() -> ("CtlRef"=w438:refnum<vi>)  [unwired: 1 in]
        n105 = property class="Bool (strict)"(reference=w438) -> ("Label.Text"=w439:string)  [unwired: 1 in, 2 out]
        n106 = call "RelayControl.vi"("Neutron Shutter"="Neutron Shutter", "Error In"=w454, "Sample Space Pump"="Sample Space Pump", "Siphon Pump"="Siphon Pump", "Relay In"=w453) -> ("Error Out"=w449:errorcluster, "Relay Out"=w450:refnum<visa-resource-name>)  [unwired: 5 in]
        n107 = case shown="\"Neutron Shutter\"" w439 {
          frame "0", Default {
          }
          frame "Neutron Shutter" {
            n108 = property on="RESTART" class="Bool (strict)"("Val(Sgnl)"=TRUE ("RESTART")) -> ()  [unwired: 2 in, 2 out]
          }
        }
      }
      event "Enable": Value Change {
        n109 = event-data() -> ("OldVal"=w457:bool, "NewVal"=w458:bool)  [unwired: 1 in, 4 out]
        n110 = Not Equal?(x=w457, y=w458) -> (x != y?=w456:bool)
        n111 = case shown="True" w456 {
          tunnel: w462 -> [w472 w476]
          tunnel: w461 -> [w471 w475]
          tunnel: [w471 w474] -> w460
          tunnel: [w472 w473] -> w459
          frame False {
          }
          frame True {
            n112 = call "ToggleShutter.vi"("error in"=w475, "VISA resource name"=w476) -> ("error out"=w474:errorcluster, "VISA resource name out"=w473:refnum<visa-resource-name>)  [unwired: 8 in]
          }
        }
      }
      event "Shutter Mode": Value Change {
        n113 = event-data() -> ()  [unwired: 1 in, 6 out]
        n114 = call "ThorlabsMode.vi"("error in"=w488, "Mode"="Shutter Mode", "VISA resource name"=w489) -> ("error out"=w487:errorcluster, "VISA resource name out"=w486:refnum<visa-resource-name>)  [unwired: 7 in]
      }
      event "New Background Frame": Value Change {
        n115 = event-data() -> ("NewVal"=w492:bool)  [unwired: 1 in]
        n116 = And(x=w492, y=w491) -> (x .and. y?=w490:bool)
        n117 = case shown="True" w490 {
          tunnel: w504 -> [w505 w517]
          tunnel: w503 -> [w506 w518]
          tunnel: [w506 w515] -> w502
          tunnel: [w505 w509] -> w501
          frame False {
          }
          frame True {
            n118 = local read "Cycle time\n(ms)"() -> (w507:i32)
            n119 = local read "On CCD Acc."() -> (w516:i32)
            n120 = local read "MODE"() -> (w512:u16)
            n121 = local read "File Exists"() -> (w508:bool)
            n122 = local read "BIN"() -> (w511:u16)
            n123 = call "LightFieldAcquireBackground.vi"("Cycle time\n(ms)"=w507, "File Exists"=w508, "On CCD Acc."=w516, "error in"=w517, "BIN"=w511, "MODE"=w512, "VISA resource name"=w518) -> ("error out"=w514:errorcluster, "VISA resource name out"=w513:refnum<visa-resource-name>)  [unwired: 3 in]
            n124 = call "PGResetCameraWait.vi"("Cycle time\n(ms)"=w507, "error in"=w514, "BIN"=w511, "MODE"=w512, "VISA resource name"=w513) -> ("error out"=w510:errorcluster, "VISA resource name out"=w515:refnum<visa-resource-name>)  [unwired: 5 in]
            n125 = flat-sequence {
              tunnel: w510 -> [w520]
              tunnel: [w520] -> w509
              frame #0 {
                n126 = local write "New Background Frame"(FALSE ("New Background")) -> ()
                n127 = local write "File Exists"(TRUE ("File Exists")) -> ()
              }
            }
          }
        }
      }
      event "New Background Movie": Value Change {
        n128 = event-data() -> ("NewVal"=w532:bool)  [unwired: 1 in]
        n129 = case shown="True" w532 {
          frame False {
          }
          frame True {
            n130 = flat-sequence {
              tunnel: [w552] -> w543
              tunnel: w542 -> [w551]
              tunnel: [w551] -> w541
              tunnel: [w550] -> w540
              tunnel: w537 -> [w549]
              tunnel: [w549] -> w536
              tunnel: w543 -> [w556]
              tunnel: w541 -> [w557]
              tunnel: w540 -> [w554]
              tunnel: [w556] -> w539
              tunnel: [w554] -> w538
              tunnel: w536 -> [w553]
              tunnel: [w553] -> w535
              tunnel: w539 -> [w563]
              tunnel: w538 -> [w562]
              tunnel: w535 -> [w560]
              tunnel: [w563] -> w534
              tunnel: [w562] -> w533
              tunnel: w534 -> [w564]
              tunnel: w533 -> [w565]
              frame #0 {
                n131 = local read "Manual Script Entry (0)"() -> (w552:string)
                n132 = local read "Script\n#"() -> (w550:i32)
                n133 = Wait (ms)(milliseconds to wait=u32 15) -> ()  [unwired: 1 out]
              }
              frame #1 {
                n134 = local write "Manual Script Entry (0)"(w557) -> ()
                n135 = local write "Script\n#"(0 ("Script\n#")) -> ()
              }
              frame #2 {
                n136 = Add(x=w560, y=50) -> (x+y=w558:i32)
                n137 = property on="SCRIPTING" class="Bool (strict)"("Val(Sgnl)"=TRUE ("Value (Signaling)")) -> ()  [unwired: 2 in, 2 out]
                n138 = Wait (ms)(milliseconds to wait=w558) -> ()  [unwired: 1 out]
              }
              frame #3 {
                n139 = local write "Manual Script Entry (0)"(w564) -> ()
                n140 = local write "Script\n#"(w565) -> ()
              }
              frame #4 {
                n141 = local write "New Background Movie"(FALSE ("New Background Movie")) -> ()
              }
            }
            n142 = local read "Cycle time\n(ms)"() -> (w546:i32)
            n143 = local read "# Frames"() -> (w545:i32)
            n144 = local read "MODE"() -> (w544:u16)
            n145 = local read "BIN"() -> (w547:u16)
            n146 = call "BGScriptGenerator.vi"("Cycle time\n(ms)"=w546, "# Frames"=w545, "BIN"=w547, "MODE"=w544) -> ("Duration (ms)"=w537:i32, "BG Script"=w542:string)  [unwired: 6 in]
          }
        }
      }
    }
  }
  n147 = while {
    shift-right: [w665] -> w142
    shift-left: w141 -> [w664]
    shift-right: [w666] -> w143
    shift-left: w140 -> [w663]
    shift-right: [w660] -> w133
    shift-left: w138 -> [w662]
    shift-right: [w659] -> w132
    shift-left: w137 -> [w661]
    shift-right: [w658] -> w78
    shift-left: _ -> [w656]
    shift-right: [w657] -> w77
    shift-left: _ -> [w655]
    shift-right: [w652] -> w102
    shift-left: w113 -> [w654]
    shift-right: [w651] -> w104
    shift-left: w114 -> [w650]
    shift-right: [w648] -> w117
    shift-left: w127 -> [w649]
    shift-right: [w646] -> w118
    shift-left: w126 -> [w647]
    tunnel: w115 -> [w653]
    tunnel: [w622] -> w103
    shift-right: [w619] -> w82
    shift-left: w84 -> [w621]
    shift-right: [w618] -> w81
    shift-left: w83 -> [w620]
    shift-right: [w607] -> _
    shift-left: _ -> [w611]
    shift-right: [w606] -> w45
    shift-left: w43 -> [w603]
    shift-right: [w605] -> w46
    shift-left: w44 -> [w604]
    shift-right: [w597] -> w37
    shift-left: w41 -> [w600]
    shift-right: [w598] -> w36
    shift-left: w40 -> [w599]
    shift-right: [w591] -> _
    shift-left: _ -> [w593]
    shift-right: [w575] -> _
    shift-left: w21 -> [w577]
    shift-right: [w572] -> w12
    shift-left: w15 -> [w573]
    shift-right: [w571] -> w13
    shift-left: w16 -> [w574]
    stop <- w612 stop-if-true
    n148 = local read "DATA"() -> (w617:bool)
    n149 = Get Date/Time In Seconds() -> (seconds since 1Jan1904=w579:timestamp)
    n150 = call "Collect Data.vi"("Location of FieldMax2Lib.dll in"=w620, "Meter ID in"=w621) -> ("Location of FieldMax2Lib.dll out"=w618:path, "Meter ID out"=w619:i32, "Measurement"=w615:sgl)  [unwired: 5 in, 1 out]
    n151 = Multiply(x="Data Interval (s)", y=u32 1000 ("millisecond multiple")) -> (x*y=w623:dbl)
    n152 = To Double Precision Float(number=w579) -> (double precision float=w575:dbl)
    n153 = Subtract(x=w575, y=w577) -> (x-y=w576:dbl)
    n154 = Multiply(x=w615, y=1000.0) -> (x*y=w614:dbl)
    "Power (mW)" <- w614
    n155 = Get Date/Time String(seconds (now)=w579, want seconds? (F)=TRUE) -> (time string=→"time string":string)  [unwired: 1 in, 1 out]
    n156 = call "Lakeshore218ReadTemp.vi"("error in"=w574, "VISA resource name"=w573) -> ("error out"=w571:errorcluster, "Thick Film R (Ohms)"=w570:string, "VISA resource name out"=w572:refnum<visa-resource-name>)  [unwired: 7 in]
    n157 = case shown="True" "RECORD" {
      tunnel: w656 -> [w718 _]
      tunnel: w655 -> [w719 _]
      tunnel: [w719 w724] -> w626
      tunnel: [w718 w723] -> w627
      frame False {
      }
      frame True {
        n158 = local read "SCRIPTING"() -> (w722:bool)
        n159 = local read "Script\n#"() -> (w721:i32)
        n160 = local write "RECORD"(FALSE ("RECORD")) -> ()
        n161 = call "DataHeader.vi"("Script #"=w721, "Scripting"=w722) -> ("error out"=w723:errorcluster, "Timestamp"=→"Timestamp":string, "refnum out"=w724:refnum<file>)  [unwired: 7 in]
      }
    }
    n162 = call "Lakeshore218Parse.vi"("Resistance String"=w570) -> ("Low Level (Ohms)"=w567:dbl, "High Level (Ohms)"=→"High Level\n(Ohms)":dbl)  [unwired: 9 in]
    "Low Level\n(Ohms)" <- w567
    n163 = call-poly "Open.vi"("error in (no error)"=w663, "Device Identifier"="MB1.T1:TEMP", "Mercury Reference In"=w664) -> ("error out"=w639:errorcluster, "Mercury Reference Out"=w638:T4)  [unwired: 7 in]
    n164 = call-poly "Signals (Read).vi"("error in"=w639, "Mercury Reference In"=w638) -> ("error out"=w636:errorcluster, "Temperature"=w587:dbl, "Mercury Reference Out"=w637:T4)  [unwired: 5 in, 2 out]
    "Cryostat (K)" <- w587
    n165 = call-poly "Open.vi"("error in (no error)"=w636, "Device Identifier"="DB6.T1:TEMP", "Mercury Reference In"=w637) -> ("error out"=w634:errorcluster, "Mercury Reference Out"=w635:T4)  [unwired: 7 in]
    n166 = case shown="True" "AUTOFILL" {
      tunnel: w567 -> [_ w667]
      frame False {
      }
      frame True {
        n167 = Less?(x=w667, y="LL (Ohms)") -> (x < y?=w669:bool)
        n168 = case shown="True" w669 {
          selector: w669 -> [_ w670]
          frame False {
          }
          frame True {
            n169 = property on="REFILL" class="Bool (strict)"("Val(Sgnl)"=w670) -> ()  [unwired: 2 in, 2 out]
          }
        }
      }
    }
    n170 = call "PressureControl - 3He.vi"("error in (no error)"=w649, "VISA resource name"=w647) -> ("error out"=w648:errorcluster, "3HePressure (Torr)"=w581:string, "VISA resource name out"=w646:refnum<visa-resource-name>)  [unwired: 7 in]
    n171 = call "PressureControl - 4He.vi"("error in (no error)"=w662, "VISA resource name"=w661) -> ("error out"=w660:errorcluster, "Pressure"=w629:dbl, "Pressure (Torr)"=w582:string, "VISA resource name out"=w659:refnum<visa-resource-name>)  [unwired: 6 in]
    n172 = call-poly "Signals (Read).vi"("error in"=w634, "Mercury Reference In"=w635) -> ("error out"=w666:errorcluster, "Temperature"=w628:dbl, "Mercury Reference Out"=w665:T4)  [unwired: 5 in, 2 out]
    "Cell (K)" <- w628
    n173 = case shown="\"Fill Tanks\"" "Turbulence" {
      tunnel: w582 -> [w726 w729]
      tunnel: w581 -> [w727 w728]
      frame "Main Controls", Default {
        "Tank Pressure 2 (Torr)" <- w727
        "Tank Pressure 1 (Torr)" <- w726
      }
      frame "Fill Tanks" {
        n174 = event shown="[2] \"3He Pressure (Torr)\": Value Change" {
          selector: _ -> [_ _ _ _]
          dyn-events: _ -> [_ _ _ _]
          timeout: 500 ("Numeric") -> [_ _ _ _]
          tunnel: w728 -> [_ _ _ w735]
          tunnel: w729 -> [_ _ _ w737]
          event Timeout {
            n175 = event-data() -> ()  [unwired: 1 in, 3 out]
          }
          event "Desired Tank\nPressure (3He)": Value Change {
            n176 = event-data() -> ("NewVal"=w731:dbl)  [unwired: 1 in]
            n177 = call "3HePressureCalculator.vi"("Desired Tank\nPressure (3He)"=w731) -> ("V2 Pressure (3He)"=→"Desired V2\nPressure (3He)":dbl)  [unwired: 10 in]
          }
          event "3He Pressure (Torr)": Value Change {
            n178 = event-data() -> ("NewVal"=w733:string)  [unwired: 1 in]
            n179 = call "3HeActualPressure.vi"("3He Pressure (Torr)"=w733) -> ("Actual 3He\nTank Pressure"=→"Actual 3He\nTank Pressure":dbl)  [unwired: 10 in]
          }
          event "Log Pressure": Value Change {
            n180 = event-data() -> ("NewVal"=w736:bool)  [unwired: 1 in]
            n181 = call "SaveTankData.vi"("Log Pressure"=w736, "4He Pressure (Torr)"=w737, "3He Pressure (Torr)"=w735) -> ()  [unwired: 8 in]
          }
        }
        "3He Pressure (Torr)" <- w728
        "4He Pressure (Torr)" <- w729
      }
    }
    n182 = call-poly "DAQmx Read.vi"("task/channels in"=w604, "error in"=w603) -> ("task out"=w602:refnum<k21>, "data"=w607:dbl, "error out"=w601:errorcluster)  [unwired: 11 in]
    "Detected" <- w607
    n183 = call-poly "DAQmx Read.vi"("task/channels in"=w600, "error in"=w599) -> ("task out"=w596:refnum<k21>, "data"=w591:dbl, "error out"=w595:errorcluster)  [unwired: 11 in]
    "Incident" <- w591
    n184 = case shown="True" w617 {
      tunnel: w650 -> [w677 w707]
      tunnel: w654 -> [w679 w706]
      tunnel: w653 -> [w678 w705]
      tunnel: [w678 w701] -> w633
      tunnel: [w677 w700] -> w632
      tunnel: [w679 w699] -> w631
      tunnel: w628 -> [_ w693]
      tunnel: w587 -> [_ w691]
      tunnel: w627 -> [w675 w690]
      tunnel: w582 -> [_ w689]
      tunnel: w626 -> [w676 w688]
      tunnel: [w675 w687] -> w625
      tunnel: [w676 w686] -> w624
      tunnel: w623 -> [w674 w684]
      tunnel: [w674 w683] -> w613
      tunnel: w614 -> [_ w682]
      tunnel: w607 -> [_ w681]
      tunnel: w591 -> [_ w680]
      frame False {
      }
      frame True {
        n185 = Subtract(x=w684, y=350.0) -> (x-y=w683:dbl)
        n186 = call "Measure.vi"("Function (Current)"=T6."Power", "error in (no error)"=w707, "Node In"=w705, "VISA resource name"=w706) -> ("error out"=w698:errorcluster, "Output"=w692:string, "Node Out"=w702:string, "VISA resource name out"=w703:refnum<visa-resource-name>)  [unwired: 3 in, 1 out]
        n187 = flat-sequence {
          tunnel: w698 -> [w708]
          tunnel: [w708] -> w697
          frame #0 {
            n188 = Wait (ms)(milliseconds to wait=u32 100) -> ()  [unwired: 1 out]
          }
        }
        n189 = call "Measure.vi"("Function (Current)"=T6."Power", "error in (no error)"=w697, "Channel (Channel A)"=Channel."Channel B", "Node In"=w702, "VISA resource name"=w703) -> ("error out"=w700:errorcluster, "Output"=w694:string, "Node Out"=w701:string, "VISA resource name out"=w699:refnum<visa-resource-name>)  [unwired: 2 in, 1 out]
        n190 = call "CompileData.vi"("Detected"=w681, "Incident"=w680, "Ch. B (W)"=w694, "Cell Temp (K)"=w693, "Ch. A (W)"=w692, "Cryostat Temp (K)"=w691, "error in"=w690, "Laser Power (W)"=w682, "Tank Pressure (Torr)"=w689, "refnum in"=w688) -> ("error out"=w687:errorcluster, "refnum out"=w686:refnum<file>)
      }
    }
    n191 = case shown="True" "CLOSE" {
      tunnel: w625 -> [w710 w716]
      tunnel: w624 -> [w711 w715]
      tunnel: [w711 refnum<file> refnum ("refnum out")] -> w657
      tunnel: [w710 errorcluster {"status"=FALSE, "code"=0, "source"=""} ("error out")] -> w658
      frame False {
      }
      frame True {
        n192 = local write "CLOSE"(FALSE ("CLOSE")) -> ()
        n193 = Close File(refnum=w715, error in=w716) -> (error out=→"File I/O Error":errorcluster)  [unwired: 1 out]
      }
    }
    n194 = Less?(x=w587, y=3.0) -> (x < y?=w584:bool)
    n195 = event shown="[5] \"RESTART\": Value Change" {
      selector: _ -> [_ _ _ _ _ _]
      dyn-events: _ -> [_ _ _ _ _ _]
      timeout: w613 -> [_ _ _ _ _ _]
      tunnel: w633 -> [w742 w756 w768 w780 w792 w805]
      tunnel: w632 -> [w743 w757 w770 w782 w794 w806]
      tunnel: w631 -> [w744 w755 w767 w779 w791 w804]
      tunnel: [w744 w754 w769 w781 w793 w804] -> w652
      tunnel: [w743 w750 w763 w777 w788 w806] -> w651
      tunnel: [w742 w749 w762 w776 w787 w805] -> w622
      tunnel: [w741 w748 w761 w775 w786 w803] -> w606
      tunnel: [w740 w747 w760 w774 w785 w802] -> w605
      tunnel: w602 -> [w740 w747 w760 w774 w785 w801]
      tunnel: w601 -> [w741 w748 w761 w775 w786 w800]
      tunnel: [w739 w746 w759 w773 w784 w798] -> w597
      tunnel: [w738 w745 w758 w772 w783 w797] -> w598
      tunnel: w596 -> [w739 w746 w759 w773 w784 w796]
      tunnel: w595 -> [w738 w745 w758 w772 w783 w795]
      event Timeout {
        n196 = event-data() -> ()  [unwired: 1 in, 3 out]
      }
      event "Top Coil (mA)": Value Change {
        n197 = event-data() -> ("NewVal"=w752:dbl)  [unwired: 1 in, 5 out]
        n198 = Divide(x=w752, y=1000.0) -> (x/y=w751:dbl)
        n199 = call "Source Level.vi"("Level (0.000)"=w751, "error in (no error)"=w757, "Node In"=w756, "VISA resource name"=w755) -> ("error out"=w750:errorcluster, "Node Out"=w749:string, "VISA resource name out"=w754:refnum<visa-resource-name>)  [unwired: 4 in, 1 out]
      }
      event "Bottom Coil (mA)": Value Change {
        n200 = event-data() -> ("NewVal"=w765:dbl)  [unwired: 1 in, 5 out]
        n201 = Divide(x=w765, y=1000.0) -> (x/y=w764:dbl)
        n202 = call "Source Level.vi"("Level (0.000)"=w764, "error in (no error)"=w770, "Channel (Channel A)"=Channel."Channel B", "Node In"=w768, "VISA resource name"=w767) -> ("error out"=w763:errorcluster, "Node Out"=w762:string, "VISA resource name out"=w769:refnum<visa-resource-name>)  [unwired: 3 in, 1 out]
      }
      event "Top Coil": Value Change {
        n203 = event-data() -> ("NewVal"=w778:bool)  [unwired: 1 in, 5 out]
        n204 = call "Source Output Enable.vi"("Output (Off)"=w778, "error in (no error)"=w782, "Node In"=w780, "VISA resource name"=w779) -> ("error out"=w777:errorcluster, "Node Out"=w776:string, "VISA resource name out"=w781:refnum<visa-resource-name>)  [unwired: 4 in, 1 out]
      }
      event "Bottom Coil": Value Change {
        n205 = event-data() -> ("NewVal"=w789:bool)  [unwired: 1 in, 5 out]
        n206 = call "Source Output Enable.vi"("Output (Off)"=w789, "error in (no error)"=w794, "Channel (Channel A)"=Channel."Channel B", "Node In"=w792, "VISA resource name"=w791) -> ("error out"=w788:errorcluster, "Node Out"=w787:string, "VISA resource name out"=w793:refnum<visa-resource-name>)  [unwired: 3 in, 1 out]
      }
      event "RESTART": Value Change {
        n207 = event-data() -> ("NewVal"=w799:bool)  [unwired: 1 in, 5 out]
        n208 = case shown="True" w799 {
          tunnel: w801 -> [w810 w820]
          tunnel: w800 -> [w809 w821]
          tunnel: [w810 w819] -> w802
          tunnel: [w809 w818] -> w803
          tunnel: [w808 w814] -> w798
          tunnel: [w807 w813] -> w797
          tunnel: w796 -> [w808 w812]
          tunnel: w795 -> [w807 w811]
          frame False {
          }
          frame True {
            n209 = call "DAQmx Stop Task.vi"("task/channels in"=w820, "error in"=w821) -> ("task out"=w817:refnum<k21>, "error out"=w822:errorcluster)  [unwired: 12 in]
            n210 = call "DAQmx Stop Task.vi"("task/channels in"=w812, "error in"=w811) -> ("task out"=w815:refnum<k21>, "error out"=w816:errorcluster)  [unwired: 12 in]
            n211 = local write "RESTART"(FALSE ("RESTART")) -> ()
            n212 = call "DAQmx Start Task.vi"("task/channels in"=w817, "error in"=w822) -> ("task out"=w819:refnum<k21>, "error out"=w818:errorcluster)  [unwired: 12 in]
            n213 = call "DAQmx Start Task.vi"("task/channels in"=w815, "error in"=w816) -> ("task out"=w814:refnum<k21>, "error out"=w813:errorcluster)  [unwired: 12 in]
          }
        }
      }
    }
    n214 = Subtract(x=w591, y=w593) -> (x-y=w592:dbl)
    n215 = Subtract(x=w607, y=w611) -> (x-y=w610:dbl)
    n216 = Less?(x=w629, y=15.0) -> (x < y?=w585:bool)
    n217 = And(x=w584, y=w585) -> (x .and. y?=w583:bool)
    n218 = Divide(x=w592, y=w576) -> (x/y=→"Rate (Hz)":dbl)
    n219 = Divide(x=w610, y=w576) -> (x/y=→"Rate (Hz)":dbl)
    n220 = case shown="True" w583 {
      tunnel: [FALSE ("RUN/STOP") TRUE ("RUN/STOP")] -> w588
      frame False {
      }
      frame True {
      }
    }
    n221 = property on="READY" class="Bool (strict)"() -> ("Value"=w590:bool)  [unwired: 2 in, 2 out]
    n222 = Equal?(x=w590, y=w588) -> (x = y?=w589:bool)
    n223 = case shown="False" w589 {
      tunnel: w588 -> [w671 _]
      frame False {
        n224 = property on="READY" class="Bool (strict)"("Val(Sgnl)"=w671) -> ()  [unwired: 2 in, 2 out]
      }
      frame True {
      }
    }
    n225 = local read "Kill Switch"() -> (w612:bool)
  }
  n226 = local write "3He Check"(TRUE ("3He Check")) -> ()
  n227 = call "LogHeader.vi"("Data folder"=path "C:/Data") -> ("error out"=w73:errorcluster, "refnum out"=w74:refnum<file>)  [unwired: 9 in]
  "Log" <- w74
  n228 = call "MFCInit.vi"() -> ("MFC error out"=w8:errorcluster, "MFC VISA out"=w7:refnum<visa-resource-name>)  [unwired: 10 in]
  n229 = while {
    shift-right: [w834] -> w72
    shift-left: w74 -> [w835]
    shift-right: [w833] -> w71
    shift-left: w73 -> [w836]
    shift-right: [w827] -> w4
    shift-left: w7 -> [w831]
    shift-right: [w828] -> w5
    shift-left: w8 -> [w832]
    shift-right: [w829] -> _
    shift-left: 0.0 ("3He Pressure") -> [w830]
    stop <- w826 stop-if-true
    n230 = event shown="[0] \"SCRIPTING\": Value Change" {
      selector: _ -> [_ _ _ _]
      dyn-events: _ -> [_ _ _ _]
      timeout: 500 -> [_ _ _ _]
      tunnel: w836 -> [w844 w1326 w1399 w1413]
      tunnel: w835 -> [w845 w1325 w1400 w1414]
      tunnel: [w843 w1325 w1400 w1414] -> w834
      tunnel: [w842 w1326 w1399 w1413] -> w833
      tunnel: w832 -> [w839 w1331 w1403 w1411]
      tunnel: w831 -> [w838 w1332 w1404 w1410]
      tunnel: w830 -> [w840 w1330 w1402 w1412]
      tunnel: [w840 w1329 w1401 w1412] -> w829
      tunnel: [w839 w1328 w1403 w1411] -> w828
      tunnel: [w838 w1327 w1404 w1410] -> w827
      event "SCRIPTING": Value Change {
        n231 = event-data() -> ()  [unwired: 1 in, 1 out]
        n232 = case shown="True" "SCRIPTING" {
          tunnel: w845 -> [w847 w851]
          tunnel: w844 -> [w846 w850]
          tunnel: [w847 w848] -> w843
          tunnel: [w846 w849] -> w842
          frame False {
          }
          frame True {
            n233 = local read "Script\n#"() -> (w853:i32)
            n234 = Not Equal To 0?(x=w853) -> (x != 0?=w852:bool)
            n235 = case shown="False" w852 {
              tunnel: w851 -> [w859 w1043]
              tunnel: w850 -> [w860 w1044]
              tunnel: [w854 w1041] -> w849
              tunnel: [w855 w1042] -> w848
              frame False {
                n236 = call "GetManualCommands.vi"("Manual Script Entry (0)"="Manual Script Entry (0)") -> ("Commands"=w867:string[])  [unwired: 10 in]
                n237 = Array Size(array=w867) -> (size(s)=w863:i32)
                n238 = for {
                  tunnel: w867 -> [w899] mode=indexing
                  tunnel: [w894] -> w866
                  tunnel: [w893] -> w861
                  i -> [w894]
                  stop <- w896 stop-if-true
                  n239 = Match Pattern(string=w899, regular expression="[a-z]+") -> (match substring=w892:string, after substring=w891:string)  [unwired: 1 in, 2 out]
                  n240 = call "Trim Whitespace.vi"("string"=w891) -> ("trimmed string"=w898:string)  [unwired: 1 in]
                  n241 = Concatenate Strings(w892, w891) -> (w890:string)
                  n242 = case shown="\"data\"" w892 {
                    tunnel: w898 -> [_ w912 w931 w946 w953 w971 w989 w1018]
                    tunnel: [TRUE ("Top Coil") w911 w928 FALSE ("Top Coil") w950 w968 w988 w1017] -> w895
                    tunnel: w894 -> [w904 w910 w930 _ w952 w970 w987 w1016]
                    tunnel: u32 0 ("Script Number") -> [w903 w909 w929 _ w951 w969 w986 w1015]
                    tunnel: [w902 w907 w926 "" ("Error String") w948 w967 w984 w1013] -> w893
                    tunnel: w890 -> [w901 w906 w925 _ w947 w966 w983 w1012]
                    frame "False", Default {
                      n243 = call "ErrorHandling.vi"("Bad Command"=w901, "Line #"=w904, "Script #"=w903) -> ("Error String"=w902:string)  [unwired: 8 in]
                    }
                    frame "data" {
                      n244 = case shown="\"False\", Default" w912 {
                        tunnel: [FALSE ("DATA") TRUE ("DATA") FALSE ("DATA")] -> w908
                        tunnel: [TRUE ("Top Coil") FALSE ("Top Coil") FALSE ("Top Coil")] -> w911
                        tunnel: w910 -> [w915 _ _]
                        tunnel: w909 -> [w916 _ _]
                        tunnel: [w914 "" ("Error String") "" ("Error String")] -> w907
                        tunnel: w906 -> [w913 _ _]
                        frame "False", Default {
                          n245 = call "ErrorHandling.vi"("Bad Command"=w913, "Line #"=w915, "Script #"=w916) -> ("Error String"=w914:string)  [unwired: 8 in]
                        }
                        frame "on" {
                        }
                        frame "off" {
                        }
                      }
                      n246 = property on="DATA" class="Bool (strict)"("Val(Sgnl)"=w908) -> ()  [unwired: 2 in, 2 out]
                    }
                    frame "pulse" {
                      n247 = case shown="\"False\", Default" w931 {
                        tunnel: [FALSE ("Top Coil") TRUE ("Top Coil") w942] -> w927
                        tunnel: [TRUE FALSE w942] -> w928
                        tunnel: w930 -> [w935 _ _]
                        tunnel: w929 -> [w934 _ _]
                        tunnel: [w933 "" ""] -> w926
                        tunnel: w925 -> [w932 _ _]
                        frame "False", Default {
                          n248 = call "ErrorHandling.vi"("Bad Command"=w932, "Line #"=w935, "Script #"=w934) -> ("Error String"=w933:string)  [unwired: 8 in]
                        }
                        frame "on" {
                        }
                        frame "off" {
                          w942 = FALSE ("Top Coil")
                        }
                      }
                      n249 = property on="RUN/STOP" class="Bool (strict)"("Val(Sgnl)"=w927) -> ()  [unwired: 2 in, 2 out]
                    }
                    frame "wait" {
                      n250 = Decimal String To Number(string=w946) -> (number=w945:i32)  [unwired: 2 in, 1 out]
                      n251 = Wait (ms)(milliseconds to wait=w945) -> ()  [unwired: 1 out]
                    }
                    frame "neutron" {
                      n252 = case shown="\"False\", Default" w953 {
                        tunnel: w952 -> [w959 _ _]
                        tunnel: w951 -> [w958 _ _]
                        tunnel: [TRUE ("Top Coil") FALSE ("Top Coil") w964] -> w950
                        tunnel: [FALSE ("Neutron Shutter") TRUE ("Neutron Shutter") w964] -> w949
                        tunnel: [w955 "" ("Error String") "" ("Error String")] -> w948
                        tunnel: w947 -> [w954 _ _]
                        frame "False", Default {
                          n253 = call "ErrorHandling.vi"("Bad Command"=w954, "Line #"=w959, "Script #"=w958) -> ("Error String"=w955:string)  [unwired: 8 in]
                        }
                        frame "on" {
                        }
                        frame "off" {
                          w964 = FALSE ("Neutron Shutter")
                        }
                      }
                      n254 = property on="Neutron Shutter" class="Bool (strict)"("Val(Sgnl)"=w949) -> ()  [unwired: 2 in, 2 out]
                    }
                    frame "shutter" {
                      n255 = case shown="\"False\", Default" w971 {
                        tunnel: w970 -> [w977 _ _]
                        tunnel: w969 -> [w976 _ _]
                        tunnel: [TRUE ("Top Coil") FALSE ("Top Coil") w982] -> w968
                        tunnel: [FALSE ("Neutron Shutter") TRUE ("Neutron Shutter") w982] -> w965
                        tunnel: [w973 "" ("Error String") "" ("Error String")] -> w967
                        tunnel: w966 -> [w972 _ _]
                        frame "False", Default {
                          n256 = call "ErrorHandling.vi"("Bad Command"=w972, "Line #"=w977, "Script #"=w976) -> ("Error String"=w973:string)  [unwired: 8 in]
                        }
                        frame "on" {
                        }
                        frame "off" {
                          w982 = FALSE ("Neutron Shutter")
                        }
                      }
                      n257 = property on="Enable" class="Bool (strict)"("Val(Sgnl)"=w965) -> ()  [unwired: 2 in, 2 out]
                    }
                    frame "coila" {
                      n258 = case shown="\"False\", Default" w989 {
                        selector: w989 -> [w996 _]
                        tunnel: [w998 w1011] -> w985
                        tunnel: [w997 w1011] -> w988
                        tunnel: w987 -> [w993 _]
                        tunnel: w986 -> [w992 _]
                        tunnel: [w991 "" ("Error String")] -> w984
                        tunnel: w983 -> [w990 _]
                        frame "False", Default {
                          n259 = Match Pattern(string=w996, regular expression="[^0-9.]") -> (offset past match=w994:i32)  [unwired: 1 in, 3 out]
                          n260 = case shown="0, Default" w994 {
                            tunnel: [FALSE ("Top Coil") TRUE ("Top Coil")] -> w998
                            tunnel: [TRUE FALSE] -> w997
                            tunnel: w996 -> [_ w1007]
                            tunnel: w993 -> [w1002 _]
                            tunnel: w992 -> [w1001 _]
                            tunnel: [w1000 ""] -> w991
                            tunnel: w990 -> [w999 _]
                            frame 0, Default {
                              n261 = call "ErrorHandling.vi"("Bad Command"=w999, "Line #"=w1002, "Script #"=w1001) -> ("Error String"=w1000:string)  [unwired: 8 in]
                            }
                            frame -1 {
                              n262 = Fract/Exp String To Number(string=w1007) -> (number=w1006:dbl)  [unwired: 3 in, 1 out]
                              n263 = property on="Top Coil (mA)" class="DigNum (strict)"("Val(Sgnl)"=w1006) -> ()  [unwired: 2 in, 2 out]
                            }
                          }
                        }
                        frame "off" {
                          w1011 = FALSE ("Top Coil")
                        }
                      }
                      n264 = property on="Top Coil" class="Bool (strict)"("Val(Sgnl)"=w985) -> ()  [unwired: 2 in, 2 out]
                    }
                    frame "coilb" {
                      n265 = case shown="\"False\", Default" w1018 {
                        selector: w1018 -> [w1025 _]
                        tunnel: [w1024 w1040] -> w1014
                        tunnel: [w1023 w1040] -> w1017
                        tunnel: w1016 -> [w1022 _]
                        tunnel: w1015 -> [w1021 _]
                        tunnel: [w1020 ""] -> w1013
                        tunnel: w1012 -> [w1019 _]
                        frame "False", Default {
                          n266 = Match Pattern(string=w1025, regular expression="[^0-9.]") -> (offset past match=w1026:i32)  [unwired: 1 in, 3 out]
                          n267 = case shown="0, Default" w1026 {
                            tunnel: w1025 -> [_ w1038]
                            tunnel: [FALSE TRUE] -> w1024
                            tunnel: [TRUE FALSE] -> w1023
                            tunnel: w1022 -> [w1031 _]
                            tunnel: w1021 -> [w1030 _]
                            tunnel: [w1029 ""] -> w1020
                            tunnel: w1019 -> [w1028 _]
                            frame 0, Default {
                              n268 = call "ErrorHandling.vi"("Bad Command"=w1028, "Line #"=w1031, "Script #"=w1030) -> ("Error String"=w1029:string)  [unwired: 8 in]
                            }
                            frame -1 {
                              n269 = Fract/Exp String To Number(string=w1038) -> (number=w1035:dbl)  [unwired: 3 in, 1 out]
                              n270 = property on="Bottom Coil (mA)" class="DigNum (strict)"("Val(Sgnl)"=w1035) -> ()  [unwired: 2 in, 2 out]
                            }
                          }
                        }
                        frame "off" {
                          w1040 = FALSE
                        }
                      }
                      n271 = property on="Bottom Coil" class="Bool (strict)"("Val(Sgnl)"=w1014) -> ()  [unwired: 2 in, 2 out]
                    }
                  }
                  n272 = local read "Kill Switch"() -> (w889:bool)
                  n273 = Or(x=w895, y=w889) -> (x .or. y?=w896:bool)
                }
                n274 = Decrement(x=w863) -> (x-1=w865:i32)
                n275 = Equal?(x=w866, y=w865) -> (x = y?=w864:bool)
                n276 = case shown="False" w864 {
                  tunnel: [w883 w886] -> w862
                  tunnel: w861 -> [w881 _]
                  tunnel: [w879 w885] -> w857
                  frame False {
                    w878 = FALSE ("status")
                    n277 = property on="Bottom Coil" class="Bool (strict)"("Val(Sgnl)"=w878) -> ()  [unwired: 2 in, 2 out]
                    n278 = property on="Neutron Shutter" class="Bool (strict)"("Val(Sgnl)"=w878) -> ()  [unwired: 2 in, 2 out]
                    n279 = property on="Top Coil" class="Bool (strict)"("Val(Sgnl)"=w878) -> ()  [unwired: 2 in, 2 out]
                    n280 = property on="Enable" class="Bool (strict)"("Val(Sgnl)"=w878) -> ()  [unwired: 2 in, 2 out]
                    n281 = property on="RUN/STOP" class="Bool (strict)"("Val(Sgnl)"=w878) -> ()  [unwired: 2 in, 2 out]
                    n282 = property on="DATA" class="Bool (strict)"("Val(Sgnl)"=w878) -> ()  [unwired: 2 in, 2 out]
                    n283 = Concatenate Strings("Manual test failed!" ("Description"), "\r\n", w881) -> (w879:string)
                    n284 = Bundle("status"=w878, "code"=1017, w879) -> (w883:cluster{"status":bool, "code":i32, string})  [unwired: 1 in]
                  }
                  frame True {
                    w885 = "Manual test successful!" ("Description")
                    n285 = Bundle("status"=FALSE, "code"=0, "Description"=w885) -> (w886:T2)  [unwired: 1 in]
                  }
                }
                n286 = flat-sequence {
                  tunnel: w862 -> [w875]
                  tunnel: w860 -> [w871]
                  tunnel: w859 -> [w874]
                  tunnel: "Manual Script Entry (0)" -> [w873]
                  tunnel: w857 -> [w872]
                  tunnel: [w870] -> w856
                  tunnel: [w869] -> w854
                  tunnel: w856 -> [w877]
                  tunnel: [w877] -> w855
                  frame #0 {
                    n287 = local write "Scripting \nError"(w875) -> ()
                    n288 = local read "Timestamp"() -> (w868:string)
                    n289 = call "WriteResults_Manual.vi"("Timestamp"=w868, "error in"=w871, "Result"=w872, "Commands"=w873, "refnum in"=w874) -> ("error out"=w869:errorcluster, "refnum out"=w870:refnum<file>)  [unwired: 5 in]
                  }
                  frame #1 {
                    n290 = property on="SCRIPTING" class="Bool (strict)"("Val(Sgnl)"=FALSE ("Value (Signaling)")) -> ()  [unwired: 2 in, 2 out]
                  }
                }
              }
              frame True {
                n291 = while {
                  tunnel: w1044 -> [w1050]
                  tunnel: w1043 -> [w1049]
                  tunnel: [w1048] -> w1042
                  tunnel: [w1046] -> w1041
                  stop <- w1045 stop-if-true
                  n292 = local read "Script\n#"() -> (w1052:i32)
                  n293 = call "GetCommands.vi"("Script Number"=w1052) -> ("Script Exists"=w1053:bool, "Commands"=w1054:string[], "Camera Settings"=w1055:dbl[], "Data Interval (s)"=w1051:dbl)  [unwired: 5 in]
                  n294 = case shown="True" w1053 {
                    tunnel: w1055 -> [_ w1093]
                    tunnel: w1054 -> [_ w1091]
                    tunnel: w1052 -> [w1072 w1089]
                    tunnel: w1051 -> [_ w1088]
                    tunnel: w1050 -> [w1066 w1086]
                    tunnel: w1049 -> [w1067 w1085]
                    tunnel: [w1065 w1084] -> w1048
                    tunnel: [w1064 w1083] -> w1047
                    frame False {
                      n295 = Number To Decimal String(number=w1072) -> (decimal integer string=w1071:string)  [unwired: 1 in]
                      n296 = Concatenate Strings("Script" ("string"), w1071, " does not exist." ("string")) -> (w1068:string)
                      n297 = Bundle("status"=FALSE, "code"=1017, w1068) -> (w1073:cluster{"status":bool, "code":i32, string})  [unwired: 1 in]
                      n298 = Get Date/Time In Seconds() -> (seconds since 1Jan1904=w1063:timestamp)
                      n299 = Format Date/Time String(time format string (%c)="%H:%M:%S", seconds (now)=w1063) -> (date/time string=w1061:string)  [unwired: 1 in]
                      n300 = local write "Scripting \nError"(w1073) -> ()
                      n301 = call "WriteResults_Script.vi"("Timestamp"=w1061, "error in"=w1066, "Result"=w1068, "refnum in"=w1067) -> ("error out"=w1064:errorcluster, "refnum out"=w1065:refnum<file>)  [unwired: 6 in]
                      n302 = property on="SCRIPTING" class="Bool (strict)"("Val(Sgnl)"=FALSE ("Value (Signaling)")) -> ()  [unwired: 2 in, 2 out]
                    }
                    frame True {
                      n303 = flat-sequence {
                        tunnel: u32 100 ("milliseconds to wait") -> [w1102]
                        tunnel: w1093 -> [w1103]
                        tunnel: [w1103] -> w1082
                        tunnel: [w1102] -> w1081
                        tunnel: w1088 -> [w1101]
                        tunnel: w1082 -> [w1107]
                        tunnel: [w1107] -> w1100
                        tunnel: w1081 -> [w1106]
                        tunnel: [w1106] -> w1099
                        tunnel: w1100 -> [w1112]
                        tunnel: [w1112] -> w1098
                        tunnel: w1099 -> [w1111]
                        tunnel: [w1111] -> w1097
                        tunnel: w1098 -> [w1116]
                        tunnel: [w1116] -> w1080
                        tunnel: w1097 -> [w1115]
                        tunnel: [w1115] -> w1079
                        tunnel: w1080 -> [w1120]
                        tunnel: w1079 -> [w1121]
                        tunnel: [w1121] -> w1078
                        tunnel: [w1120] -> w1077
                        tunnel: [w1124] -> w1096
                        tunnel: w1078 -> [w1123]
                        tunnel: [w1123] -> w1095
                        tunnel: w1077 -> [w1124]
                        tunnel: w1096 -> [w1129]
                        tunnel: w1095 -> [w1128]
                        tunnel: w1091 -> [w1134]
                        tunnel: w1089 -> [w1133]
                        tunnel: [w1132] -> w1094
                        tunnel: [w1131] -> w1087
                        tunnel: w1090 -> [w1297]
                        tunnel: w1094 -> [w1298]
                        tunnel: w1089 -> [w1287]
                        tunnel: w1087 -> [w1294]
                        tunnel: w1086 -> [w1291]
                        tunnel: w1085 -> [w1292]
                        tunnel: [w1290] -> w1084
                        tunnel: [w1289] -> w1083
                        frame #0 {
                          n304 = property on="Data Interval (s)" class="DigNum (strict)"("Val(Sgnl)"=w1101) -> ()  [unwired: 2 in, 2 out]
                        }
                        frame #1 {
                          n305 = Index Array(array=w1107, index=0) -> (element=w1105:dbl)
                          n306 = To Unsigned Word Integer(number=w1105) -> (unsigned 16bit integer=w1104:u16)
                          n307 = local write "MODE"(w1104) -> ()
                        }
                        frame #2 {
                          n308 = Index Array(array=w1112, index=1) -> (element=w1110:dbl)
                          n309 = To Unsigned Word Integer(number=w1110) -> (unsigned 16bit integer=w1109:u16)
                          n310 = local write "BIN"(w1109) -> ()
                        }
                        frame #3 {
                          n311 = Index Array(array=w1116, index=2) -> (element=w1114:dbl)
                          n312 = local write "On CCD Acc."(w1114) -> ()
                        }
                        frame #4 {
                          n313 = Index Array(array=w1120, index=3) -> (element=w1118:dbl)
                          n314 = local write "Cycle time\n(ms)"(w1118) -> ()
                        }
                        frame #5 {
                          n315 = Index Array(array=w1124, index=4) -> (element=w1122:dbl)
                          n316 = property on="# Frames" class="DigNum (strict)"("Val(Sgnl)"=w1122) -> ()  [unwired: 2 in, 2 out]
                          n317 = Wait (ms)(milliseconds to wait=w1123) -> ()  [unwired: 1 out]
                        }
                        frame #6 {
                          n318 = Index Array(array=w1129, index=5) -> (element=w1127:dbl)
                          n319 = To Unsigned Word Integer(number=w1127) -> (unsigned 16bit integer=w1126:u16)
                          n320 = property on="Shutter Mode" class="Ring (strict)"("Val(Sgnl)"=w1126) -> ()  [unwired: 2 in, 2 out]
                          n321 = Wait (ms)(milliseconds to wait=w1128) -> ()  [unwired: 1 out]
                        }
                        frame #7 {
                          n322 = for {
                            tunnel: w1134 -> [w1146] mode=indexing
                            tunnel: w1133 -> [w1143]
                            tunnel: [w1140] -> w1132
                            tunnel: [w1139] -> w1131
                            i -> [w1140]
                            stop <- w1135 stop-if-true
                            n323 = Match Pattern(string=w1146, regular expression="[a-z]+") -> (match substring=w1138:string, after substring=w1137:string)  [unwired: 1 in, 2 out]
                            n324 = call "Trim Whitespace.vi"("string"=w1137) -> ("trimmed string"=w1144:string)  [unwired: 1 in]
                            n325 = Concatenate Strings(w1138, w1137) -> (w1136:string)
                            n326 = case shown="\"data\"" w1138 {
                              tunnel: w1144 -> [_ w1158 w1177 w1192 w1199 w1217 w1235 w1264]
                              tunnel: [TRUE ("Top Coil") w1157 w1174 FALSE ("Top Coil") w1196 w1214 w1234 w1263] -> w1142
                              tunnel: w1140 -> [w1150 w1156 w1176 _ w1198 w1216 w1233 w1262]
                              tunnel: w1143 -> [w1149 w1155 w1175 _ w1197 w1215 w1232 w1261]
                              tunnel: [w1147 w1153 w1172 "" ("Error String") w1194 w1213 w1230 w1259] -> w1139
                              tunnel: w1136 -> [w1148 w1152 w1171 _ w1193 w1212 w1229 w1258]
                              frame "False", Default {
                                n327 = call "ErrorHandling.vi"("Bad Command"=w1148, "Line #"=w1150, "Script #"=w1149) -> ("Error String"=w1147:string)  [unwired: 8 in]
                              }
                              frame "data" {
                                n328 = case shown="\"False\", Default" w1158 {
                                tunnel: [FALSE ("DATA") TRUE ("DATA") FALSE ("DATA")] -> w1154
                                tunnel: [TRUE ("Top Coil") FALSE ("Top Coil") FALSE ("Top Coil")] -> w1157
                                tunnel: w1156 -> [w1161 _ _]
                                tunnel: w1155 -> [w1162 _ _]
                                tunnel: [w1160 "" ""] -> w1153
                                tunnel: w1152 -> [w1159 _ _]
                                frame "False", Default {
                                n329 = call "ErrorHandling.vi"("Bad Command"=w1159, "Line #"=w1161, "Script #"=w1162) -> ("Error String"=w1160:string)  [unwired: 8 in]
                                }
                                frame "on" {
                                }
                                frame "off" {
                                }
                                }
                                n330 = property on="DATA" class="Bool (strict)"("Val(Sgnl)"=w1154) -> ()  [unwired: 2 in, 2 out]
                              }
                              frame "pulse" {
                                n331 = case shown="\"False\", Default" w1177 {
                                tunnel: [FALSE ("Top Coil") TRUE ("Top Coil") w1188] -> w1173
                                tunnel: [TRUE FALSE w1188] -> w1174
                                tunnel: w1176 -> [w1181 _ _]
                                tunnel: w1175 -> [w1180 _ _]
                                tunnel: [w1179 "" ("Error String") ""] -> w1172
                                tunnel: w1171 -> [w1178 _ _]
                                frame "False", Default {
                                n332 = call "ErrorHandling.vi"("Bad Command"=w1178, "Line #"=w1181, "Script #"=w1180) -> ("Error String"=w1179:string)  [unwired: 8 in]
                                }
                                frame "on" {
                                }
                                frame "off" {
                                w1188 = FALSE ("Top Coil")
                                }
                                }
                                n333 = property on="RUN/STOP" class="Bool (strict)"("Val(Sgnl)"=w1173) -> ()  [unwired: 2 in, 2 out]
                              }
                              frame "wait" {
                                n334 = Decimal String To Number(string=w1192) -> (number=w1191:i32)  [unwired: 2 in, 1 out]
                                n335 = Wait (ms)(milliseconds to wait=w1191) -> ()  [unwired: 1 out]
                              }
                              frame "neutron" {
                                n336 = case shown="\"on\"" w1199 {
                                tunnel: w1198 -> [w1205 _ _]
                                tunnel: w1197 -> [w1204 _ _]
                                tunnel: [TRUE ("Top Coil") FALSE ("Top Coil") w1210] -> w1196
                                tunnel: [FALSE ("Neutron Shutter") TRUE ("Neutron Shutter") w1210] -> w1195
                                tunnel: [w1201 "" ""] -> w1194
                                tunnel: w1193 -> [w1200 _ _]
                                frame "False", Default {
                                n337 = call "ErrorHandling.vi"("Bad Command"=w1200, "Line #"=w1205, "Script #"=w1204) -> ("Error String"=w1201:string)  [unwired: 8 in]
                                }
                                frame "on" {
                                }
                                frame "off" {
                                w1210 = FALSE ("Neutron Shutter")
                                }
                                }
                                n338 = property on="Neutron Shutter" class="Bool (strict)"("Val(Sgnl)"=w1195) -> ()  [unwired: 2 in, 2 out]
                              }
                              frame "shutter" {
                                n339 = case shown="\"off\"" w1217 {
                                tunnel: w1216 -> [w1223 _ _]
                                tunnel: w1215 -> [w1222 _ _]
                                tunnel: [TRUE ("Top Coil") FALSE ("Top Coil") w1228] -> w1214
                                tunnel: [FALSE ("Neutron Shutter") TRUE ("Neutron Shutter") w1228] -> w1211
                                tunnel: [w1219 "" ""] -> w1213
                                tunnel: w1212 -> [w1218 _ _]
                                frame "False", Default {
                                n340 = call "ErrorHandling.vi"("Bad Command"=w1218, "Line #"=w1223, "Script #"=w1222) -> ("Error String"=w1219:string)  [unwired: 8 in]
                                }
                                frame "on" {
                                }
                                frame "off" {
                                w1228 = FALSE ("Neutron Shutter")
                                }
                                }
                                n341 = property on="Enable" class="Bool (strict)"("Val(Sgnl)"=w1211) -> ()  [unwired: 2 in, 2 out]
                              }
                              frame "coila" {
                                n342 = case shown="\"False\", Default" w1235 {
                                selector: w1235 -> [w1242 _]
                                tunnel: [w1244 w1257] -> w1231
                                tunnel: [w1243 w1257] -> w1234
                                tunnel: w1233 -> [w1239 _]
                                tunnel: w1232 -> [w1238 _]
                                tunnel: [w1237 ""] -> w1230
                                tunnel: w1229 -> [w1236 _]
                                frame "False", Default {
                                n343 = Match Pattern(string=w1242, regular expression="[^0-9.]") -> (offset past match=w1240:i32)  [unwired: 1 in, 3 out]
                                n344 = case shown="-1" w1240 {
                                tunnel: [FALSE ("Top Coil") TRUE ("Top Coil")] -> w1244
                                tunnel: [TRUE FALSE] -> w1243
                                tunnel: w1242 -> [_ w1253]
                                tunnel: w1239 -> [w1248 _]
                                tunnel: w1238 -> [w1247 _]
                                tunnel: [w1246 ""] -> w1237
                                tunnel: w1236 -> [w1245 _]
                                frame 0, Default {
                                n345 = call "ErrorHandling.vi"("Bad Command"=w1245, "Line #"=w1248, "Script #"=w1247) -> ("Error String"=w1246:string)  [unwired: 8 in]
                                }
                                frame -1 {
                                n346 = Fract/Exp String To Number(string=w1253) -> (number=w1252:dbl)  [unwired: 3 in, 1 out]
                                n347 = property on="Top Coil (mA)" class="DigNum (strict)"("Val(Sgnl)"=w1252) -> ()  [unwired: 2 in, 2 out]
                                }
                                }
                                }
                                frame "off" {
                                w1257 = FALSE ("Top Coil")
                                }
                                }
                                n348 = property on="Top Coil" class="Bool (strict)"("Val(Sgnl)"=w1231) -> ()  [unwired: 2 in, 2 out]
                              }
                              frame "coilb" {
                                n349 = case shown="\"off\"" w1264 {
                                selector: w1264 -> [w1271 _]
                                tunnel: [w1270 w1286] -> w1260
                                tunnel: [w1269 w1286] -> w1263
                                tunnel: w1262 -> [w1268 _]
                                tunnel: w1261 -> [w1267 _]
                                tunnel: [w1266 "" ("Error String")] -> w1259
                                tunnel: w1258 -> [w1265 _]
                                frame "False", Default {
                                n350 = Match Pattern(string=w1271, regular expression="[^0-9.]") -> (offset past match=w1272:i32)  [unwired: 1 in, 3 out]
                                n351 = case shown="-1" w1272 {
                                tunnel: w1271 -> [_ w1284]
                                tunnel: [FALSE TRUE] -> w1270
                                tunnel: [TRUE FALSE] -> w1269
                                tunnel: w1268 -> [w1277 _]
                                tunnel: w1267 -> [w1276 _]
                                tunnel: [w1275 ""] -> w1266
                                tunnel: w1265 -> [w1274 _]
                                frame 0, Default {
                                n352 = call "ErrorHandling.vi"("Bad Command"=w1274, "Line #"=w1277, "Script #"=w1276) -> ("Error String"=w1275:string)  [unwired: 8 in]
                                }
                                frame -1 {
                                n353 = Fract/Exp String To Number(string=w1284) -> (number=w1281:dbl)  [unwired: 3 in, 1 out]
                                n354 = property on="Bottom Coil (mA)" class="DigNum (strict)"("Val(Sgnl)"=w1281) -> ()  [unwired: 2 in, 2 out]
                                }
                                }
                                }
                                frame "off" {
                                w1286 = FALSE
                                }
                                }
                                n355 = property on="Bottom Coil" class="Bool (strict)"("Val(Sgnl)"=w1260) -> ()  [unwired: 2 in, 2 out]
                              }
                            }
                            n356 = local read "Kill Switch"() -> (w1141:bool)
                            n357 = Or(x=w1142, y=w1141) -> (x .or. y?=w1135:bool)
                          }
                        }
                        frame #8 {
                          n358 = Decrement(x=w1297) -> (x-1=w1296:i32)
                          n359 = Equal?(x=w1298, y=w1296) -> (x = y?=w1299:bool)
                          n360 = case shown="True" w1299 {
                            tunnel: w1287 -> [w1308 w1313]
                            tunnel: [w1307 w1320] -> w1295
                            tunnel: w1294 -> [w1303 _]
                            tunnel: [w1301 w1314] -> w1293
                            frame False {
                              w1300 = FALSE ("Value (Signaling)")
                              n361 = Number To Decimal String(number=w1308) -> (decimal integer string=w1305:string)  [unwired: 1 in]
                              n362 = property on="Top Coil" class="Bool (strict)"("Val(Sgnl)"=w1300) -> ()  [unwired: 2 in, 2 out]
                              n363 = property on="Bottom Coil" class="Bool (strict)"("Val(Sgnl)"=w1300) -> ()  [unwired: 2 in, 2 out]
                              n364 = property on="SCRIPTING" class="Bool (strict)"("Val(Sgnl)"=w1300) -> ()  [unwired: 2 in, 2 out]
                              n365 = property on="Neutron Shutter" class="Bool (strict)"("Val(Sgnl)"=w1300) -> ()  [unwired: 2 in, 2 out]
                              n366 = property on="DATA" class="Bool (strict)"("Val(Sgnl)"=w1300) -> ()  [unwired: 2 in, 2 out]
                              n367 = property on="RUN/STOP" class="Bool (strict)"("Val(Sgnl)"=w1300) -> ()  [unwired: 2 in, 2 out]
                              n368 = Concatenate Strings("Script" ("string"), w1305, " failed!" ("string"), "\r\n", w1303) -> (w1301:string)
                              n369 = Bundle(FALSE, 1017, w1301) -> (w1307:errorcluster)  [unwired: 1 in]
                              n370 = property on="Enable" class="Bool (strict)"("Val(Sgnl)"=w1300) -> ()  [unwired: 2 in, 2 out]
                            }
                            frame True {
                              n371 = Number To Decimal String(number=w1313) -> (decimal integer string=w1316:string)  [unwired: 1 in]
                              n372 = Less?(x=w1313, y="Script\nEnd") -> (x < y?=w1311:bool)
                              n373 = case shown="False" w1311 {
                                tunnel: w1313 -> [_ w1323]
                                frame False {
                                n374 = property on="SCRIPTING" class="Bool (strict)"("Val(Sgnl)"=FALSE ("Value (Signaling)")) -> ()  [unwired: 2 in, 2 out]
                                }
                                frame True {
                                n375 = Increment(x=w1323) -> (x+1=w1324:i32)
                                n376 = property on="Script\n#" class="DigNum (strict)"("Val(Sgnl)"=w1324) -> ()  [unwired: 2 in, 2 out]
                                n377 = Wait (ms)(milliseconds to wait=u32 5000) -> ()  [unwired: 1 out]
                                }
                              }
                              n378 = Concatenate Strings("Script" ("string"), w1316, " successful!" ("string")) -> (w1314:string)
                              n379 = Bundle(FALSE, 0, w1314) -> (w1320:errorcluster)  [unwired: 1 in]
                            }
                          }
                          "Scripting \nError" <- w1295
                          n380 = local read "Timestamp"() -> (w1288:string)
                          n381 = call "WriteResults_Script.vi"("Timestamp"=w1288, "error in"=w1291, "Result"=w1293, "refnum in"=w1292) -> ("error out"=w1289:errorcluster, "refnum out"=w1290:refnum<file>)  [unwired: 6 in]
                        }
                      }
                      n382 = Array Size(array=w1091) -> (size(s)=w1090:i32)
                    }
                  }
                  n383 = flat-sequence {
                    tunnel: w1047 -> [w1058]
                    tunnel: [w1058] -> w1046
                    tunnel: [w1057] -> w1045
                    frame #0 {
                      n384 = local read "SCRIPTING"() -> (w1059:bool)
                      n385 = local read "Kill Switch"() -> (w1056:bool)
                      n386 = Not(x=w1059) -> (.not. x?=w1060:bool)
                      n387 = Or(x=w1060, y=w1056) -> (x .or. y?=w1057:bool)
                    }
                  }
                }
              }
            }
          }
        }
      }
      event "Fill": Value Change {
        n388 = event-data() -> ("NewVal"=w1333:bool)  [unwired: 1 in]
        n389 = case shown="True" w1333 {
          tunnel: w1331 -> [w1340 w1367]
          tunnel: w1332 -> [w1339 w1366]
          tunnel: [w1338 w1365] -> w1327
          tunnel: [w1337 w1364] -> w1328
          tunnel: w1330 -> [w1336 w1355]
          tunnel: [w1336 w1355] -> w1329
          frame False {
            n390 = flat-sequence {
              tunnel: w1340 -> [w1345]
              tunnel: w1339 -> [w1344]
              tunnel: [w1343] -> w1335
              tunnel: [w1342] -> w1334
              tunnel: [w1347] -> w1337
              tunnel: [w1348] -> w1338
              tunnel: w1335 -> [w1348]
              tunnel: w1334 -> [w1347]
              frame #0 {
                n391 = call "MFCSetpoint.vi"("MFC error in"=w1345, "MFC setpoint"=0.0, "MFC VISA in"=w1344) -> ("MFC error out"=w1342:errorcluster, "MFC VISA out"=w1343:refnum<visa-resource-name>)  [unwired: 7 in]
              }
              frame #1 {
                n392 = local write "3He Check"(TRUE ("3He Check")) -> ()
              }
            }
          }
          frame True {
            n393 = local read "Desired V2\nPressure (3He)"() -> (w1354:dbl)
            n394 = flat-sequence {
              tunnel: w1349 -> [w1369]
              tunnel: w1357 -> [w1370]
              tunnel: w1366 -> [w1371]
              tunnel: w1367 -> [w1372]
              tunnel: [w1372] -> w1353
              tunnel: [w1371] -> w1352
              tunnel: [w1370] -> w1351
              tunnel: [w1369] -> w1350
              tunnel: [w1376] -> w1363
              tunnel: [w1375] -> w1362
              tunnel: [w1373] -> w1359
              tunnel: w1353 -> [w1378]
              tunnel: w1352 -> [w1377]
              tunnel: w1351 -> [w1374]
              tunnel: w1350 -> [w1373]
              tunnel: w1363 -> [w1382]
              tunnel: w1362 -> [w1381]
              tunnel: [w1382] -> w1361
              tunnel: [w1381] -> w1360
              tunnel: w1359 -> [w1380]
              tunnel: w1356 -> [w1379]
              tunnel: [w1397] -> w1364
              tunnel: [w1398] -> w1365
              tunnel: w1361 -> [w1398]
              tunnel: w1360 -> [w1397]
              frame #0 {
                n395 = local write "3He Check"(FALSE ("3He Check")) -> ()
              }
              frame #1 {
                n396 = call "MFCSetpoint.vi"("MFC error in"=w1378, "MFC setpoint"=w1374, "MFC VISA in"=w1377) -> ("MFC error out"=w1375:errorcluster, "MFC VISA out"=w1376:refnum<visa-resource-name>)  [unwired: 7 in]
              }
              frame #2 {
                n397 = while {
                  tunnel: w1380 -> [w1395]
                  tunnel: w1379 -> [w1388]
                  i -> [w1391]
                  stop <- w1385 stop-if-true
                  n398 = local read "3He Pressure (Torr)"() -> (w1387:string)
                  n399 = Fract/Exp String To Number(string=w1387) -> (number=w1386:dbl)  [unwired: 3 in, 1 out]
                  n400 = Greater?(x=w1386, y=w1395) -> (0:w1394:bool)
                  n401 = Multiply(x=w1391, y=0.01) -> (x*y=w1390:dbl)
                  n402 = local read "Kill Switch"() -> (w1383:bool)
                  n403 = Greater?(x=w1390, y=w1388) -> (0:w1392:bool)
                  n404 = Or(x=w1392, y=w1394) -> (x .or. y?=w1384:bool)
                  n405 = Or(x=w1383, y=w1384) -> (x .or. y?=w1385:bool)
                  n406 = Wait (ms)(milliseconds to wait=u32 10) -> ()  [unwired: 1 out]
                }
              }
              frame #3 {
                n407 = property on="Fill" class="Bool (strict)"("Val(Sgnl)"=FALSE ("Value (Signaling)")) -> ()  [unwired: 2 in, 2 out]
              }
            }
            n408 = Add(x=w1355, y=w1354) -> (x+y=w1349:dbl)
            n409 = local read "Fill Time (s)"() -> (w1358:u32)
            n410 = call "MFCSettingCalc.vi"("Fill Time (s)"=w1358, "SetPoint"=w1354) -> ("Time (s)"=w1356:dbl, "MFC Setting"=w1357:dbl)  [unwired: 8 in]
          }
        }
      }
      event "Tare": Value Change {
        n411 = event-data() -> ("NewVal"=w1405:bool)  [unwired: 1 in]
        n412 = case shown="True" w1405 {
          tunnel: w1402 -> [w1406 _]
          tunnel: [w1406 w1407] -> w1401
          frame False {
          }
          frame True {
            n413 = local read "3He Pressure (Torr)"() -> (w1408:string)
            n414 = Fract/Exp String To Number(string=w1408) -> (number=w1407:dbl)  [unwired: 3 in, 1 out]
            n415 = local write "Tare"(FALSE ("Tare")) -> ()
          }
        }
      }
      event Timeout {
        n416 = event-data() -> ()  [unwired: 1 in, 3 out]
      }
    }
    n417 = local read "Kill Switch"() -> (w824:bool)
    n418 = And(x=w824, y="3He Check") -> (x .and. y?=w826:bool)
  }
  n419 = while {
    stop <- w1416 stop-if-true
    n420 = event shown="[2] \"REFILL\": Value Change" {
      selector: _ -> [_ _ _]
      dyn-events: _ -> [_ _ _]
      timeout: 500 -> [_ _ _]
      event Timeout {
        n421 = event-data() -> ()  [unwired: 1 in, 3 out]
      }
      event "COOLDOWN": Value Change {
        n422 = event-data() -> ("NewVal"=w1417:bool)  [unwired: 1 in, 5 out]
        n423 = case shown="True" w1417 {
          frame False {
          }
          frame True {
            n424 = flat-sequence {
              frame #0 {
                n425 = property on="Percent Open" class="DigNum (strict)"("Val(Sgnl)"=100 ("Percent Open")) -> ()  [unwired: 2 in, 2 out]
              }
              frame #1 {
                n426 = while {
                  i -> [w1422]
                  stop <- w1419 stop-if-true
                  n427 = Greater Than 0?(x=w1422) -> (x > 0?=w1421:bool)
                  n428 = case shown="True" w1421 {
                    tunnel: [FALSE ("Motor free") w1424] -> w1419
                    frame False {
                    }
                    frame True {
                      n429 = local read "Motor free"() -> (w1424:bool)
                    }
                  }
                  n430 = Wait (ms)(milliseconds to wait=u32 50) -> ()  [unwired: 1 out]
                }
              }
              frame #2 {
                n431 = property on="Sample Space Pump" class="Bool (strict)"("Val(Sgnl)"=FALSE ("Sample Space Pump")) -> ()  [unwired: 2 in, 2 out]
                n432 = Wait (ms)(milliseconds to wait=u32 100) -> ()  [unwired: 1 out]
              }
              frame #3 {
                n433 = property on="Siphon Pump" class="Bool (strict)"("Val(Sgnl)"=TRUE ("Siphon Pump")) -> ()  [unwired: 2 in, 2 out]
                n434 = Wait (ms)(milliseconds to wait=u32 100) -> ()  [unwired: 1 out]
              }
              frame #4 {
                n435 = while {
                  stop <- w1432 stop-if-true
                  n436 = local read "Kill Switch"() -> (w1435:bool)
                  n437 = local read "COOLDOWN"() -> (w1430:bool)
                  n438 = property on="Cryostat (K)" class="DigNum (strict)"() -> ("Value"=w1437:dbl)  [unwired: 2 in, 2 out]
                  n439 = Not(x=w1430) -> (.not. x?=w1429:bool)
                  n440 = Less?(x=w1437, y=3.8) -> (x < y?=w1434:bool)
                  n441 = Or(x=w1435, y=w1434) -> (x .or. y?=w1431:bool)
                  n442 = Or(x=w1431, y=w1429) -> (x .or. y?=w1432:bool)
                  n443 = Wait (ms)(milliseconds to wait=u32 1000) -> ()  [unwired: 1 out]
                }
              }
              frame #5 {
                n444 = while {
                  i -> [w1440]
                  stop <- w1439 stop-if-true
                  n445 = local read "COOLDOWN"() -> (w1445:bool)
                  n446 = local read "Kill Switch"() -> (w1442:bool)
                  n447 = Greater?(x=w1440, y="Time (s)") -> (0:w1441:bool)
                  n448 = Wait (ms)(milliseconds to wait=u32 1000) -> ()  [unwired: 1 out]
                  n449 = Not(x=w1445) -> (.not. x?=w1444:bool)
                  n450 = Or(x=w1441, y=w1442) -> (x .or. y?=w1443:bool)
                  n451 = Or(x=w1443, y=w1444) -> (x .or. y?=w1439:bool)
                }
              }
              frame #6 {
                n452 = property on="Percent Open" class="DigNum (strict)"("Val(Sgnl)"=0 ("Percent Open")) -> ()  [unwired: 2 in, 2 out]
              }
              frame #7 {
                n453 = while {
                  i -> [w1451]
                  stop <- w1448 stop-if-true
                  n454 = Greater Than 0?(x=w1451) -> (x > 0?=w1450:bool)
                  n455 = case shown="True" w1450 {
                    tunnel: [FALSE ("Motor free") w1453] -> w1448
                    frame False {
                    }
                    frame True {
                      n456 = local read "Motor free"() -> (w1453:bool)
                    }
                  }
                  n457 = Wait (ms)(milliseconds to wait=u32 50) -> ()  [unwired: 1 out]
                }
              }
              frame #8 {
                n458 = property on="Sample Space Pump" class="Bool (strict)"("Val(Sgnl)"=TRUE ("Sample Space Pump")) -> ()  [unwired: 2 in, 2 out]
                n459 = Wait (ms)(milliseconds to wait=u32 100) -> ()  [unwired: 1 out]
              }
              frame #9 {
                n460 = property on="Siphon Pump" class="Bool (strict)"("Val(Sgnl)"=FALSE ("Siphon Pump")) -> ()  [unwired: 2 in, 2 out]
                n461 = Wait (ms)(milliseconds to wait=u32 100) -> ()  [unwired: 1 out]
              }
              frame #10 {
                n462 = property on="COOLDOWN" class="Bool (strict)"("Val(Sgnl)"=FALSE ("COOLDOWN")) -> ()  [unwired: 2 in, 2 out]
              }
            }
          }
        }
      }
      event "REFILL": Value Change {
        n463 = event-data() -> ("NewVal"=w1459:bool)  [unwired: 1 in, 5 out]
        n464 = case shown="True" w1459 {
          frame False {
          }
          frame True {
            n465 = flat-sequence {
              frame #0 {
                n466 = property on="Percent Open" class="DigNum (strict)"("Val(Sgnl)"=100 ("Percent Open")) -> ()  [unwired: 2 in, 2 out]
              }
              frame #1 {
                n467 = while {
                  i -> [w1464]
                  stop <- w1461 stop-if-true
                  n468 = Greater Than 0?(x=w1464) -> (x > 0?=w1463:bool)
                  n469 = case shown="True" w1463 {
                    tunnel: [FALSE ("Motor free") w1466] -> w1461
                    frame False {
                    }
                    frame True {
                      n470 = local read "Motor free"() -> (w1466:bool)
                    }
                  }
                  n471 = Wait (ms)(milliseconds to wait=u32 50) -> ()  [unwired: 1 out]
                }
              }
              frame #2 {
                n472 = property on="Sample Space Pump" class="Bool (strict)"("Val(Sgnl)"=FALSE ("Sample Space Pump")) -> ()  [unwired: 2 in, 2 out]
                n473 = Wait (ms)(milliseconds to wait=u32 100) -> ()  [unwired: 1 out]
              }
              frame #3 {
                n474 = property on="Siphon Pump" class="Bool (strict)"("Val(Sgnl)"=TRUE ("Siphon Pump")) -> ()  [unwired: 2 in, 2 out]
                n475 = Wait (ms)(milliseconds to wait=u32 100) -> ()  [unwired: 1 out]
              }
              frame #4 {
                n476 = while {
                  stop <- w1473 stop-if-true
                  n477 = local read "High Level\n(Ohms)"() -> (w1472:dbl)
                  n478 = local read "AUTOFILL"() -> (w1478:bool)
                  n479 = local read "Kill Switch"() -> (w1475:bool)
                  n480 = Greater?(x=w1472, y="HL (Ohms)") -> (0:w1474:bool)
                  n481 = Wait (ms)(milliseconds to wait=u32 1000) -> ()  [unwired: 1 out]
                  n482 = Not(x=w1478) -> (.not. x?=w1477:bool)
                  n483 = Or(x=w1474, y=w1475) -> (x .or. y?=w1476:bool)
                  n484 = Or(x=w1476, y=w1477) -> (x .or. y?=w1473:bool)
                }
              }
              frame #5 {
                n485 = property on="Percent Open" class="DigNum (strict)"("Val(Sgnl)"=0 ("Percent Open")) -> ()  [unwired: 2 in, 2 out]
              }
              frame #6 {
                n486 = while {
                  i -> [w1484]
                  stop <- w1481 stop-if-true
                  n487 = Greater Than 0?(x=w1484) -> (x > 0?=w1483:bool)
                  n488 = case shown="True" w1483 {
                    tunnel: [FALSE ("Motor free") w1486] -> w1481
                    frame False {
                    }
                    frame True {
                      n489 = local read "Motor free"() -> (w1486:bool)
                    }
                  }
                  n490 = Wait (ms)(milliseconds to wait=u32 50) -> ()  [unwired: 1 out]
                }
              }
              frame #7 {
                n491 = property on="Sample Space Pump" class="Bool (strict)"("Val(Sgnl)"=TRUE ("Sample Space Pump")) -> ()  [unwired: 2 in, 2 out]
                n492 = Wait (ms)(milliseconds to wait=u32 100) -> ()  [unwired: 1 out]
              }
              frame #8 {
                n493 = property on="Siphon Pump" class="Bool (strict)"("Val(Sgnl)"=FALSE ("Siphon Pump")) -> ()  [unwired: 2 in, 2 out]
                n494 = Wait (ms)(milliseconds to wait=u32 100) -> ()  [unwired: 1 out]
              }
              frame #9 {
                n495 = property on="REFILL" class="Bool (strict)"("Val(Sgnl)"=FALSE ("COOLDOWN")) -> ()  [unwired: 2 in, 2 out]
              }
            }
          }
        }
      }
    }
    n496 = local read "Kill Switch"() -> (w1416:bool)
  }
  n497 = flat-sequence {
    tunnel: w28 -> [w1493]
    tunnel: [w1493] -> w27
    tunnel: [w1492] -> w26
    frame #0 {
      n498 = local read "LIGHTFIELD"() -> (w1492:bool)
    }
  }
  n499 = call "NeedleValveClose.vi"("error in (no error)"=w128, "VISA resource name"=w129) -> ("error out"=w52:errorcluster, "VISA resource name out"=w54:refnum<visa-resource-name>)  [unwired: 8 in]
  n500 = call "RelayControl.vi"("Neutron Shutter"=w76, "Error In"=w97, "Sample Space Pump"=w76, "Siphon Pump"=w76, "Relay In"=w95) -> ("Error Out"=w96:errorcluster, "Relay Out"=w94:refnum<visa-resource-name>)  [unwired: 5 in]
  n501 = flat-sequence {
    tunnel: [w1495] -> w23
    tunnel: w24 -> [w1495]
    tunnel: [w1494] -> w22
    frame #0 {
      n502 = local read "Enable"() -> (w1494:bool)
    }
  }
  n503 = flat-sequence {
    tunnel: [w1499] -> w90
    tunnel: [w1498] -> w91
    tunnel: w92 -> [w1497]
    tunnel: w93 -> [w1496]
    frame #0 {
      n504 = VISA Write(VISA resource name=w1497, write buffer=":PULSE0:STATE OFF\r\n" ("format string"), error in (no error)=w1496) -> (VISA resource name out=w1498:refnum<visa-resource-name>, error out=w1499:errorcluster)  [unwired: 1 out]
    }
  }
  n505 = VISA Close(VISA resource name=w94, error in (no error)=w96) -> (error out=w89:errorcluster)
  n506 = flat-sequence {
    tunnel: w52 -> [w1501]
    tunnel: [w1501] -> w55
    tunnel: [w1504] -> w53
    tunnel: w55 -> [w1504]
    frame #0 {
      n507 = Wait (ms)(milliseconds to wait=u32 3000) -> ()  [unwired: 1 out]
    }
    frame #1 {
      n508 = local write "Percent Open"(0 ("Percent Open")) -> ()
    }
  }
  n509 = flat-sequence {
    tunnel: w76 -> [w1505]
    tunnel: [w1506] -> w88
    tunnel: w89 -> [w1506]
    frame #0 {
      n510 = local write "Siphon Pump"(w1505) -> ()
      n511 = local write "Sample Space Pump"(w1505) -> ()
      n512 = local write "Neutron Shutter"(w1505) -> ()
    }
  }
  n513 = case shown="True" w22 {
    tunnel: [w1508 w1512] -> w33
    tunnel: [w1507 w1511] -> w32
    tunnel: w31 -> [w1507 w1510]
    tunnel: w23 -> [w1508 w1509]
    frame False {
    }
    frame True {
      n514 = call "ToggleShutter.vi"("error in"=w1509, "VISA resource name"=w1510) -> ("error out"=w1512:errorcluster, "VISA resource name out"=w1511:refnum<visa-resource-name>)  [unwired: 8 in]
    }
  }
  n515 = VISA Close(VISA resource name=w12, error in (no error)=w13) -> (error out=→"Lakeshore218 Error":errorcluster)
  n516 = Equal?(x=w26, y=TRUE) -> (x = y?=w34:bool)
  n517 = call "DAQmx Stop Task.vi"("task/channels in"=w46, "error in"=w45) -> ()  [unwired: 12 in, 2 out]
  n518 = call "DAQmx Stop Task.vi"("task/channels in"=w37, "error in"=w36) -> ()  [unwired: 12 in, 2 out]
  n519 = call "Close.vi"("error in (no error)"=w143, "Mercury Reference"=w142) -> ("error out"=w108:errorcluster)  [unwired: 9 in]
  n520 = case shown="False" w34 {
    tunnel: w35 -> [w1513 w1517]
    tunnel: w27 -> [_ w1516]
    frame False {
      n521 = local write "LightField Error"(w1513) -> ()
    }
    frame True {
      n522 = call "Adv_Deregister_for_Callback.vi"("error in (no error)"=w1517, "LightField Automation in"=w1516) -> ("error out"=w1518:errorcluster, "LightField Automation out"=w1519:refnum<class "LightField Automation.lvclass">)  [unwired: 8 in]
      n523 = call "LFA_Close.vi"("error in (no error)"=w1518, "LightField Automation in"=w1519) -> ("error out"=w1515:errorcluster)  [unwired: 8 in, 1 out]
      n524 = flat-sequence {
        tunnel: w1515 -> [w1521]
        tunnel: [w1521] -> w1514
        frame #0 {
          n525 = local write "LIGHTFIELD"(FALSE ("LIGHTFIELD")) -> ()
        }
      }
      n526 = local write "LightField Error"(w1514) -> ()
    }
  }
  n527 = call "Disconnect From Meter.vi"("Location of FieldMax2Lib.dll in"=w81, "Meter ID in"=w82) -> ()  [unwired: 7 in, 2 out]
  n528 = VISA Close(VISA resource name=w32, error in (no error)=w33) -> (error out=w30:errorcluster)
  n529 = call "KeithleyClose.vi"("Keithley Error In"=w104, "Node In"=w103, "KeithleyVISA In"=w102) -> ("Heater Error"=w101:errorcluster)  [unwired: 8 in]
  n530 = VISA Close(VISA resource name=w132, error in (no error)=w133) -> (error out=→"4He Gauge Error":errorcluster)
  n531 = call "3HeClose.vi"("error in (no error)"=w117, "VISA resource name"=w118) -> ("error out"=→"3He Gauge Error":errorcluster)  [unwired: 9 in]
  n532 = Not Equal?(x=refnum<file> refnum, y=w77) -> (x != y?=w79:bool)
  n533 = VISA Close(VISA resource name=w91, error in (no error)=w90) -> (error out=→"Pulse Generator Error":errorcluster)
  n534 = flat-sequence {
    tunnel: w101 -> [w1523]
    tunnel: [w1523] -> w100
    frame #0 {
      w1522 = FALSE ("Top Coil")
      n535 = local write "Top Coil"(w1522) -> ()
      n536 = local write "Bottom Coil"(w1522) -> ()
    }
  }
  n537 = VISA Close(VISA resource name=w54, error in (no error)=w53) -> (error out=w106:errorcluster)
  n538 = flat-sequence {
    tunnel: w30 -> [w1525]
    tunnel: [w1525] -> w29
    frame #0 {
      n539 = local write "Enable"(FALSE ("Enable")) -> ()
    }
  }
  n540 = case shown="True" w79 {
    tunnel: w78 -> [_ w1528]
    tunnel: w77 -> [_ w1527]
    frame False {
    }
    frame True {
      n541 = Close File(refnum=w1527, error in=w1528) -> (error out=w1526:errorcluster)  [unwired: 1 out]
      n542 = local write "File I/O Error"(w1526) -> ()
    }
  }
  n543 = flat-sequence {
    tunnel: w108 -> [w1534]
    tunnel: [w1534] -> w107
    tunnel: w106 -> [w1533]
    tunnel: [w1533] -> w105
    tunnel: [T2 {"status"=FALSE, "code"=0, "Description"=""} ("Scripting \nError")] -> w75
    tunnel: [w1531] -> w69
    tunnel: w70 -> [w1531]
    tunnel: w3 -> [w1529]
    tunnel: [w1529] -> w2
    frame #0 {
      w1530 = FALSE ("Kill Switch")
      n544 = local write "Kill Switch"(w1530) -> ()
      n545 = local write "READY"(w1530) -> ()
      n546 = local write "LIGHTFIELD"(w1530) -> ()
    }
  }
  n547 = local write "Scripting \nError"(w75) -> ()
  n548 = VISA Close(VISA resource name=w4, error in (no error)=w5) -> (error out=w3:errorcluster)
  n549 = Close File(refnum=w72, error in=w71) -> (error out=w70:errorcluster)  [unwired: 1 out]
  "Temperature Error" <- w107
  "Heater Error" <- w100
  "Relay Errror" <- w88
  "Zaber Motor Error" <- w105
  "Log Error" <- w69
  "Shutter Error" <- w29
  "MFC Error Out" <- w2
